vi "VolumeScan 1.4 - PointScan.vi"() -> ()   [LabVIEW 2020]
uses:
  <vilib>/vision/Image Controls.llb/IMAQ Image.ctl
  <vilib>/Utility/miscctls.llb/LVRowAndColumnTypeDef.ctl
  <vilib>/Utility/error.llb/DialogType.ctl
panel:
  out "Image":T1(plugin-control)
  in  "stop":bool
  in  "Zone":bool
  out "Status":string
  in  "Capture":bool
  in  "Tab Control":enum32{"Camera", "Display", "Saving"}(tab)
  in  "Pixels":dbl[][](array[numeric])
  in  "Threshold":dbl
  in  "Width":dbl
  in  "Band Start":dbl
  in  "ROI":dbl[](array[numeric])
  out "Node":dbl
  in  "Close camera":bool
  in  "Camera settings":bool
  in  "Camera settings table":i32(listbox)=-1
  in  "Open camera":bool
  in  "Display and panel":i32(ring) items=["2D Plot", "Default", "Graph"]
  in  "Path":path=path "G:/"
  in  "File Prefix":string="Prefix"
  in  "Save":T2(ring)
  in  "Shut Down":bool
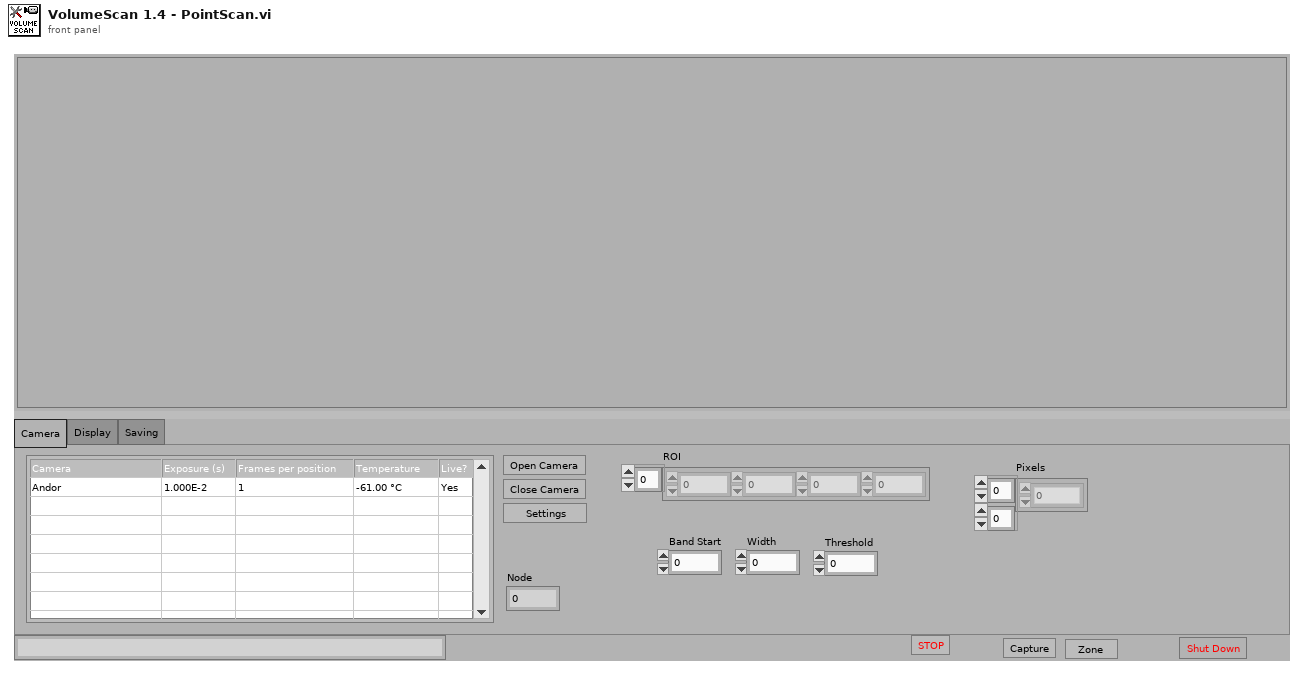
[diagram p1: front panel]
types:
  T1 = typedef "IMAQ Image.ctl" = refnum<image>
  T2 = enum16{"Don't save", "Save U16", "Save PNG", "Save TIFF"}
  T3 = cluster{"Driver":i32, "Camera settings":variant, "Update camera table":bool}
  T4 = typedef "LVRowAndColumnTypeDef.ctl" = cluster{"Row":i32, "Column":i32}
  T5 = enum8{"Enabled", "Disabled", "Disabled and Grayed Out"}
  T6 = cluster{enum16{"Image references", "Positions"}, "element data type":variant}
  T7 = enum16{"Initialize", "Shut down", "Set capture mode", "Set exposure", "Trigger and read", "Get status", "Other settings", "Idle", "Wake", "Save state"}
  T8 = enum32{"Invalid", "Standard", "Closed", "Hidden", "Minimized", "Maximized"}
  T9 = enum16{"Initialize", "Shut down", "Set capture mode", "Set exposure", "Trigger and read", "Get status", "Other settings"}
  T10 = cluster{"System OK?":bool, "Current exposure":dbl, "Temperature":dbl, "ROI":cluster{"X":u32, "X2":u32, "Y":u32, "Y2":u32}, "Binning":cluster{"X":u32, "Y":u32}}
  T11 = typedef "DialogType.ctl" = u16
  T12 = typedef "Image Type" = u32
  T13 = typedef "LVPoint32TypeDef.ctl" = cluster{"Horizontal":i32, "Vertical":i32}
  T14 = cluster{enum16{"Image references", "Positions"}, "Variant":variant}
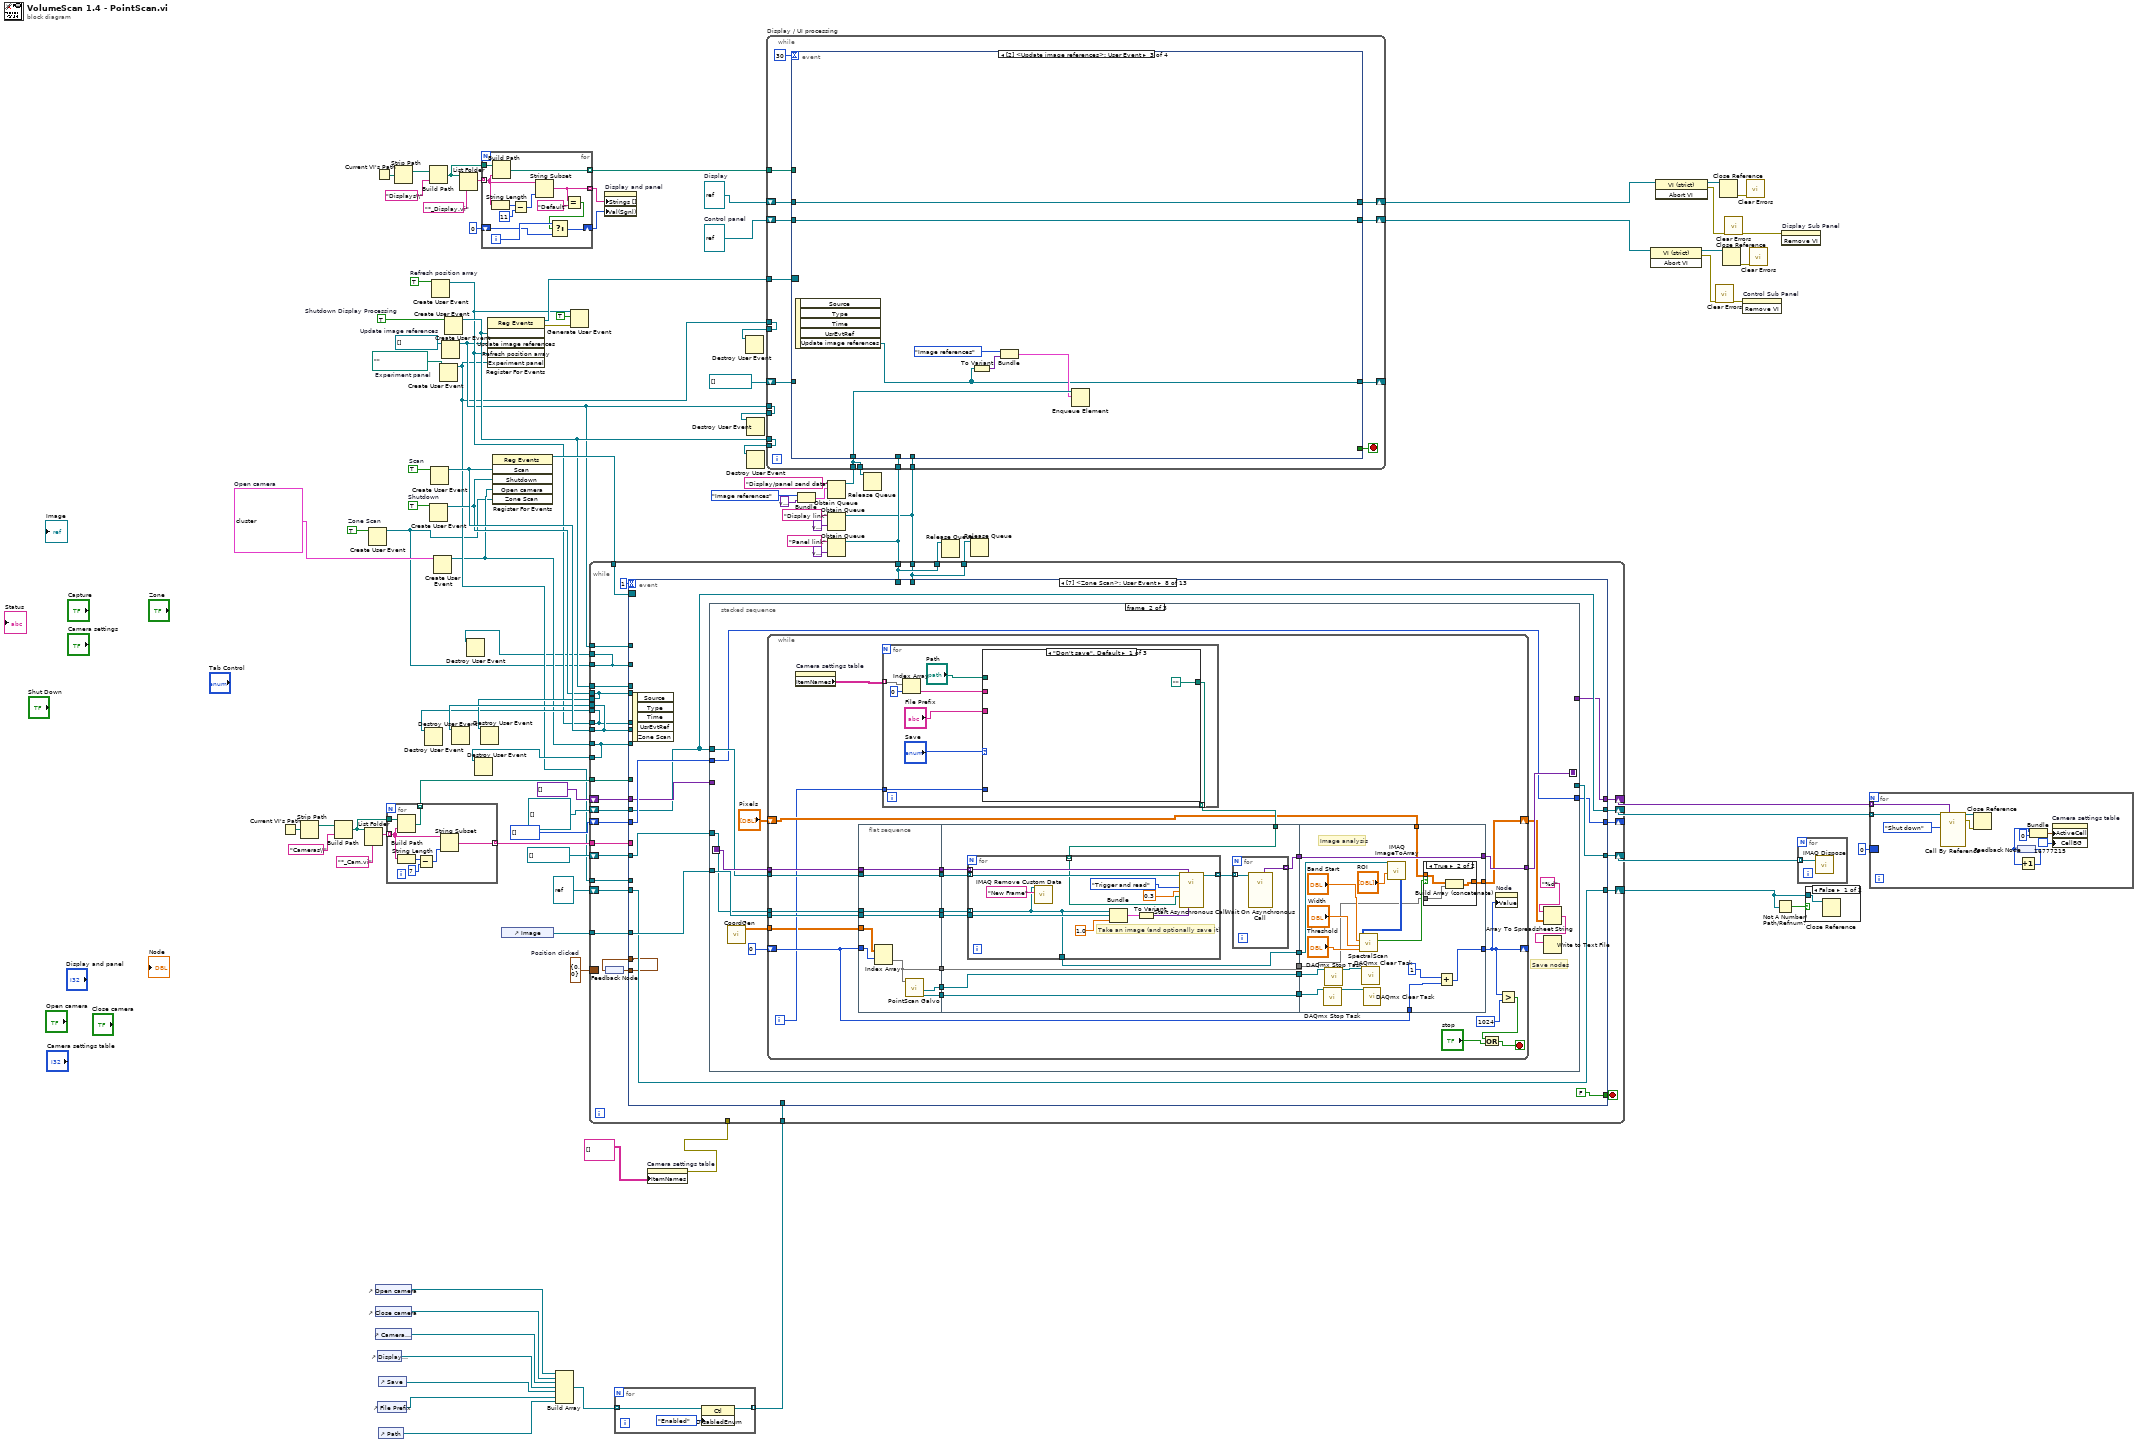
[diagram p0: block diagram]
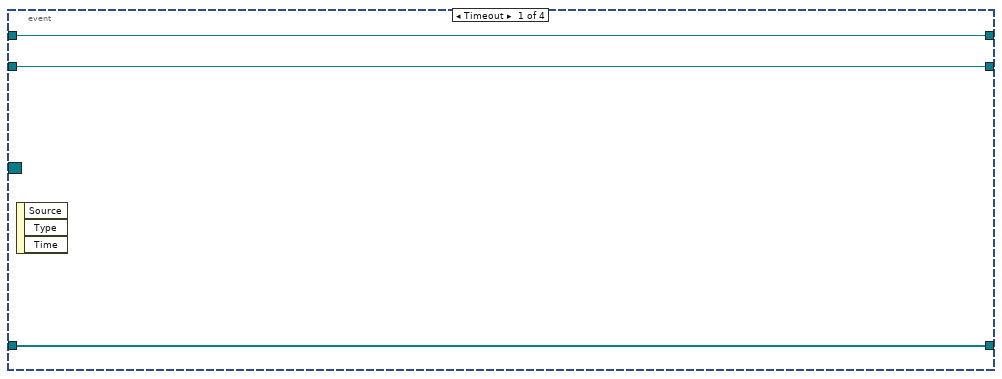
[diagram p3: hidden frame]
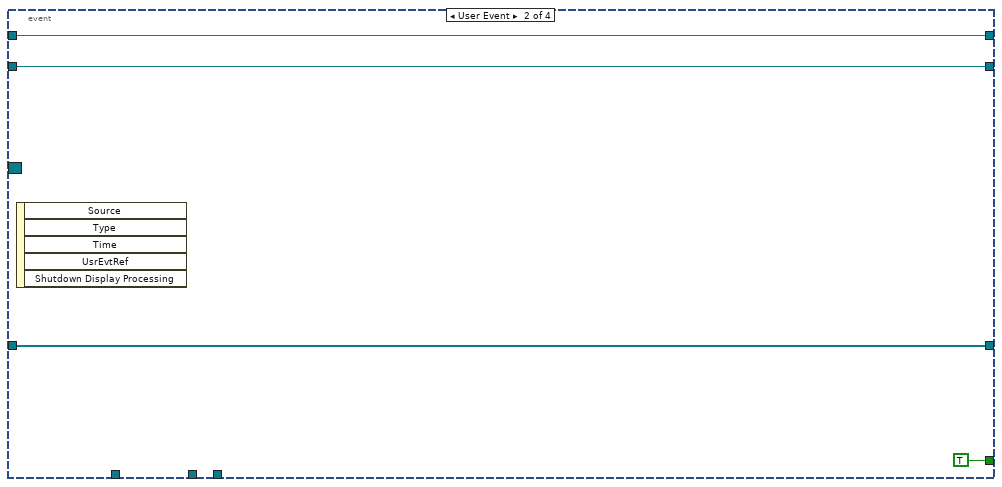
[diagram p4: hidden frame]
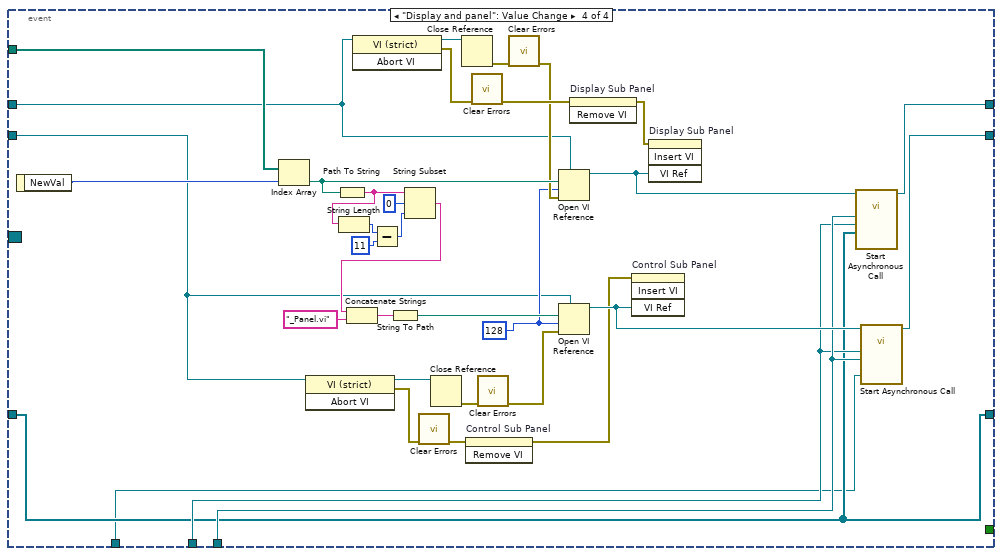
[diagram p5: hidden frame]
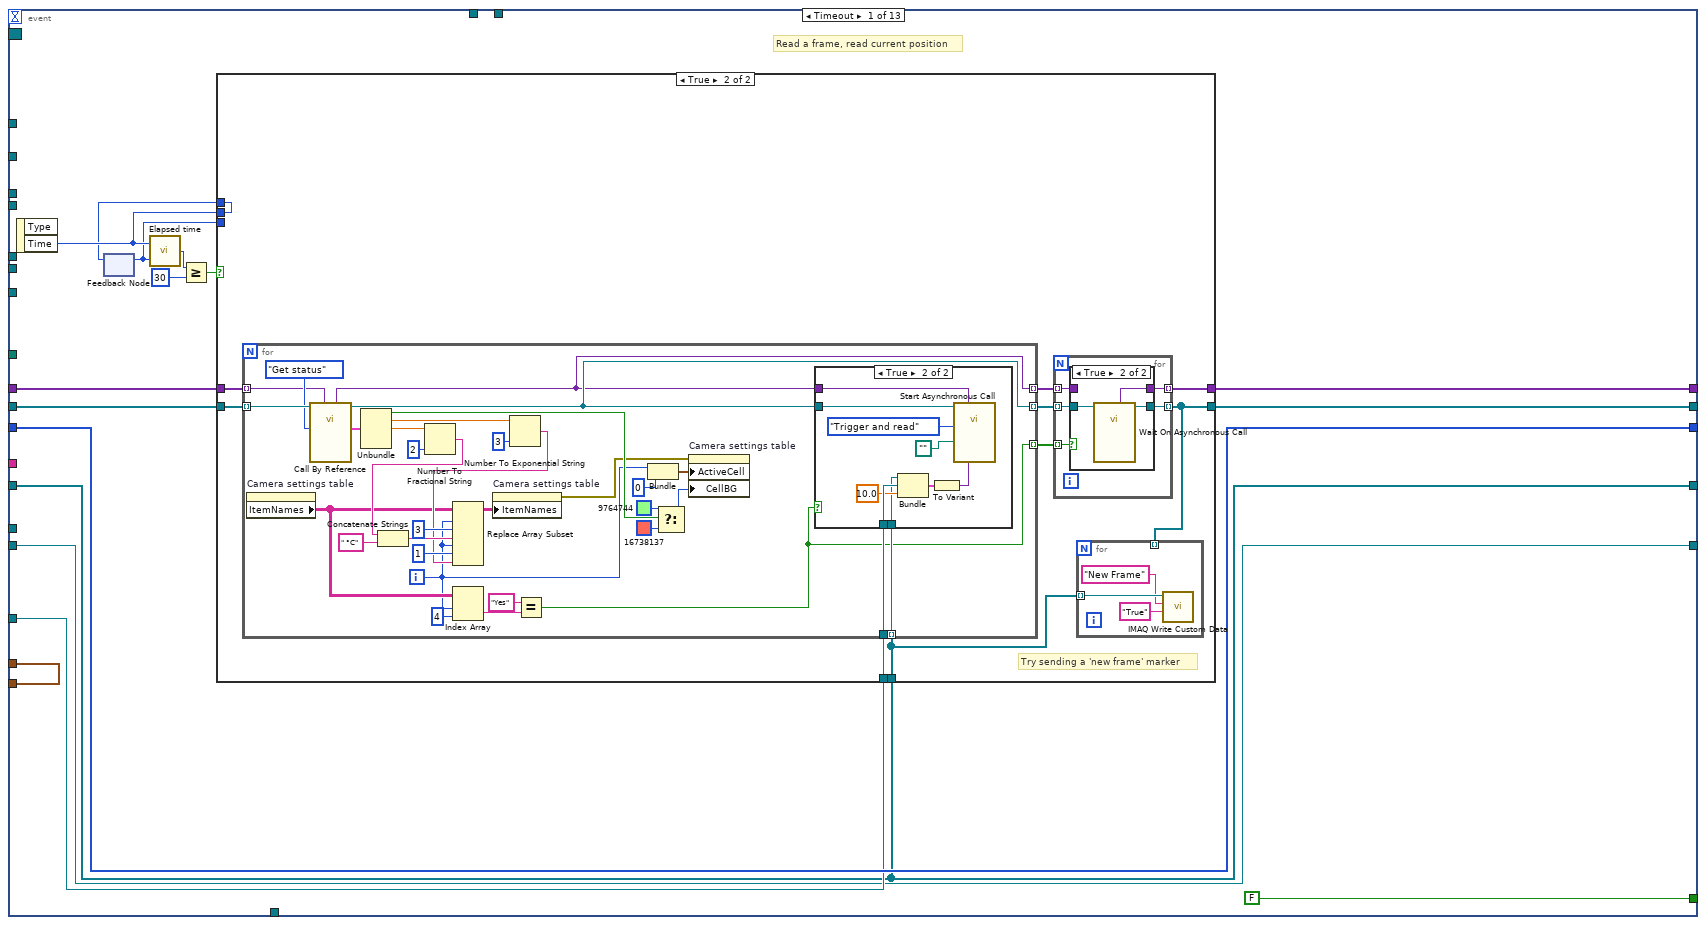
[diagram p6: hidden frame]
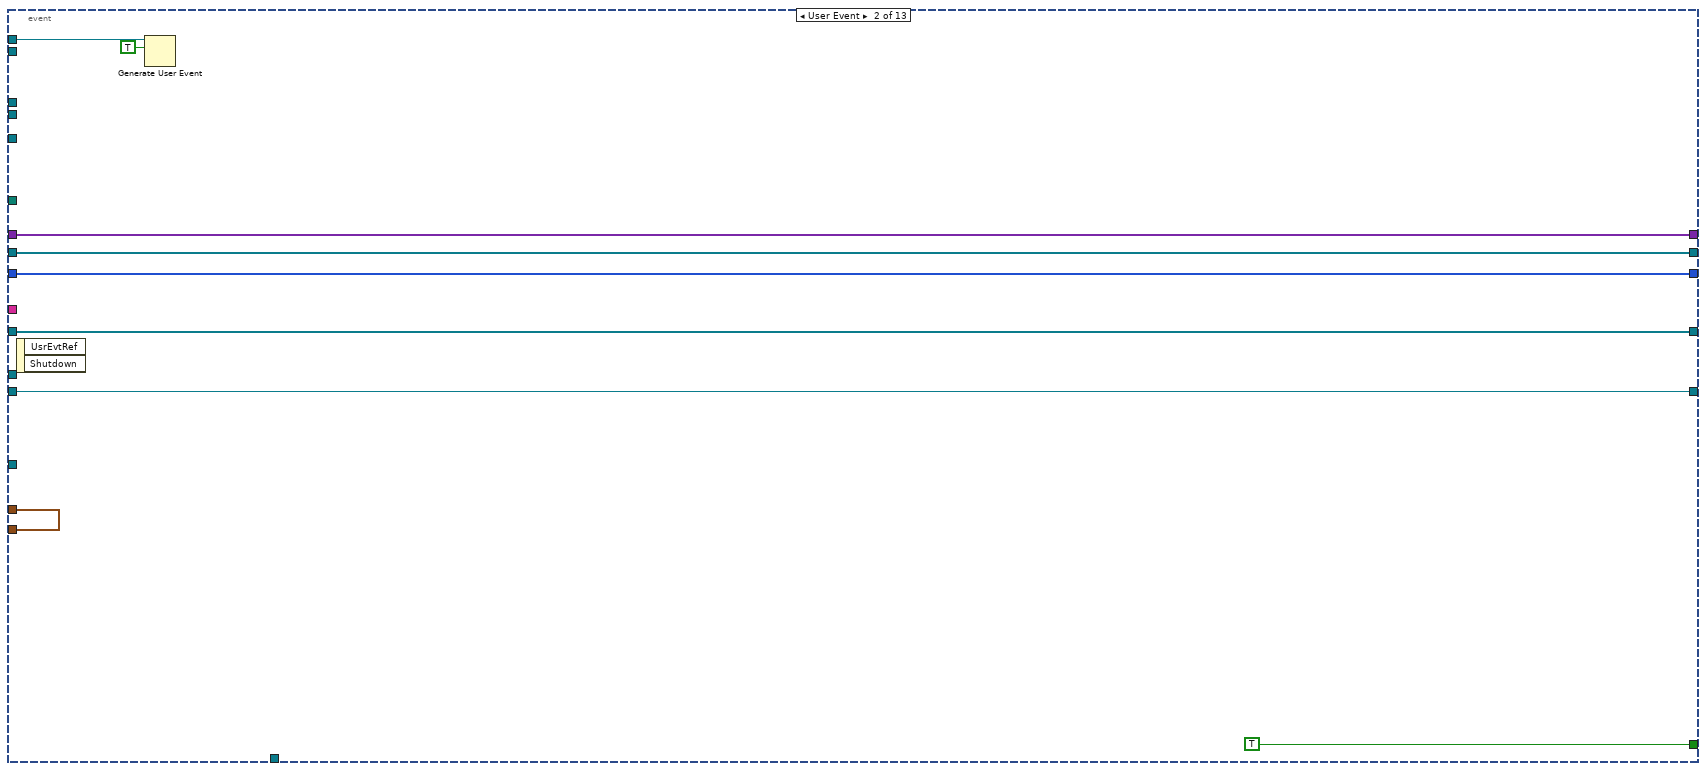
[diagram p10: hidden frame]
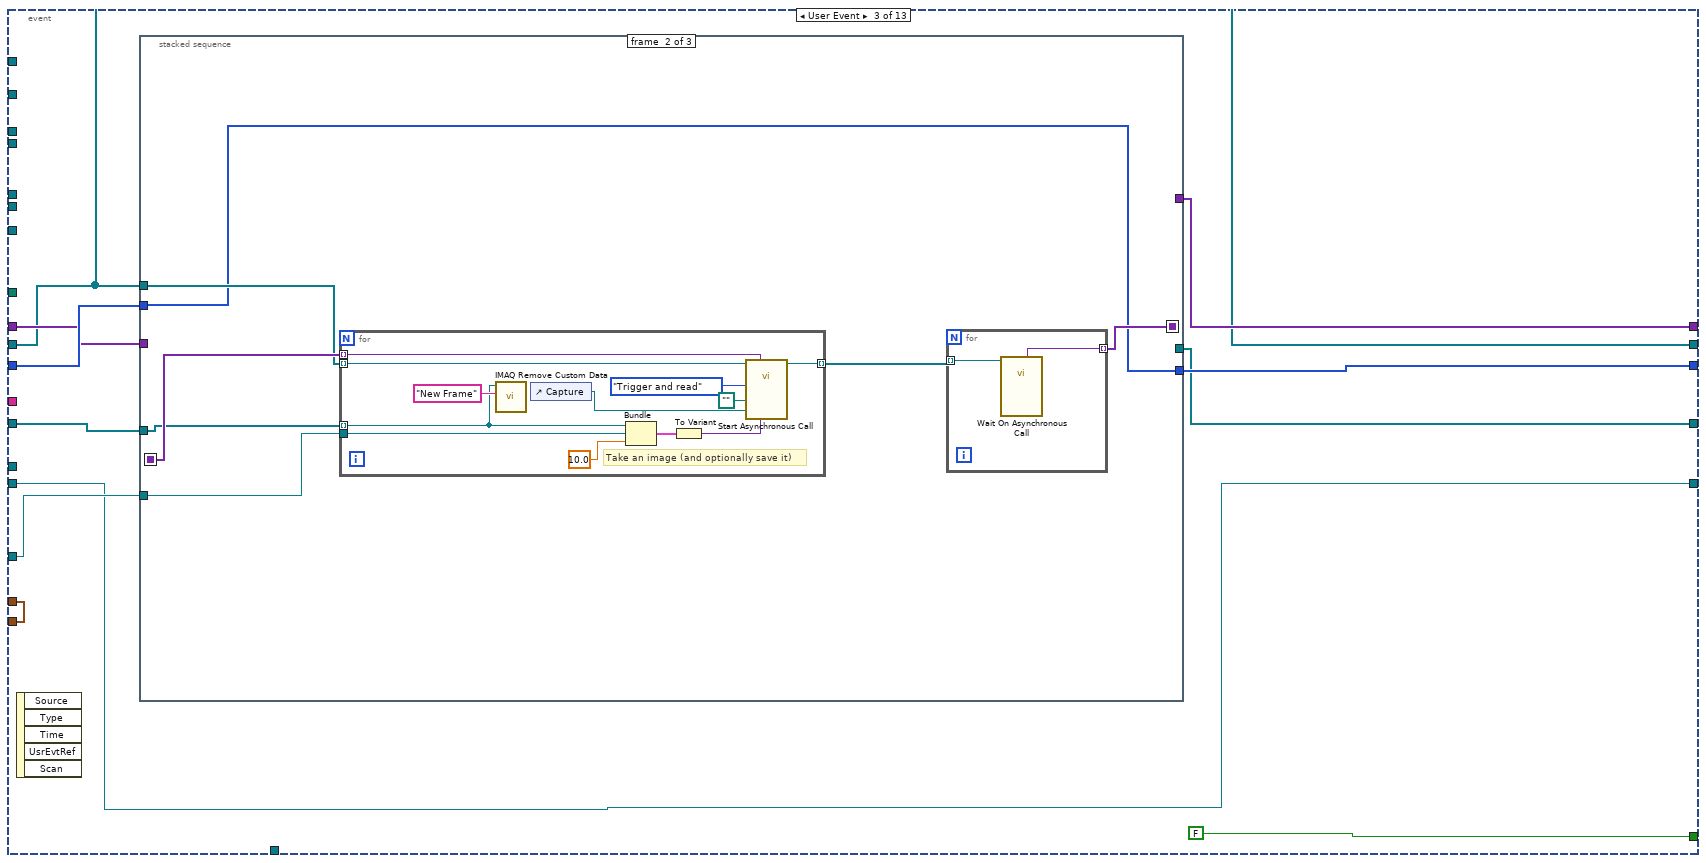
[diagram p11: hidden frame]
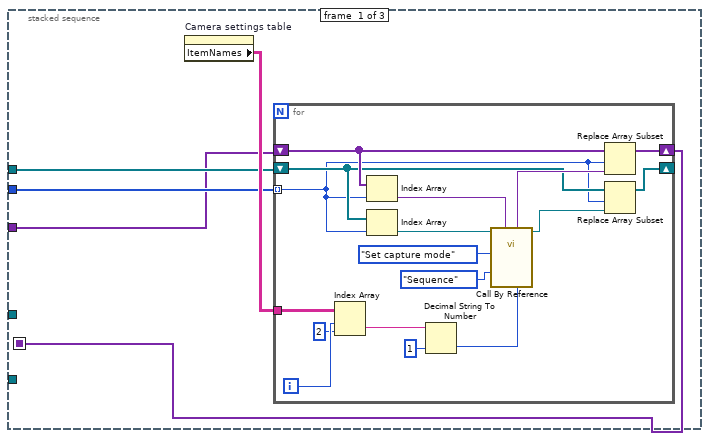
[diagram p12: hidden frame]
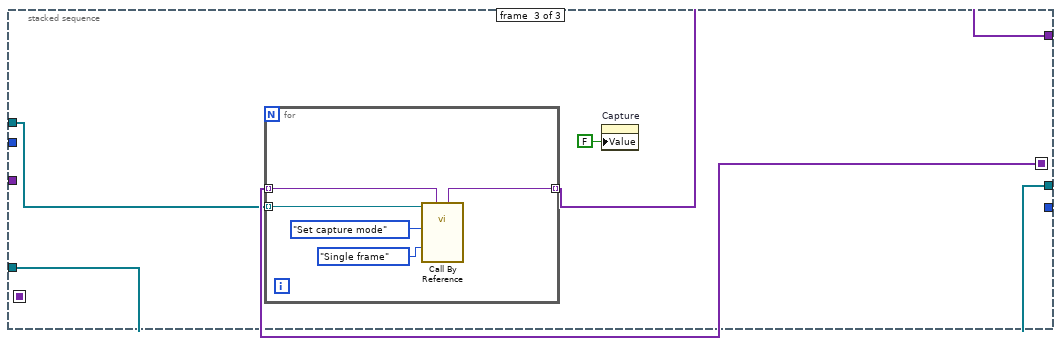
[diagram p13: hidden frame]
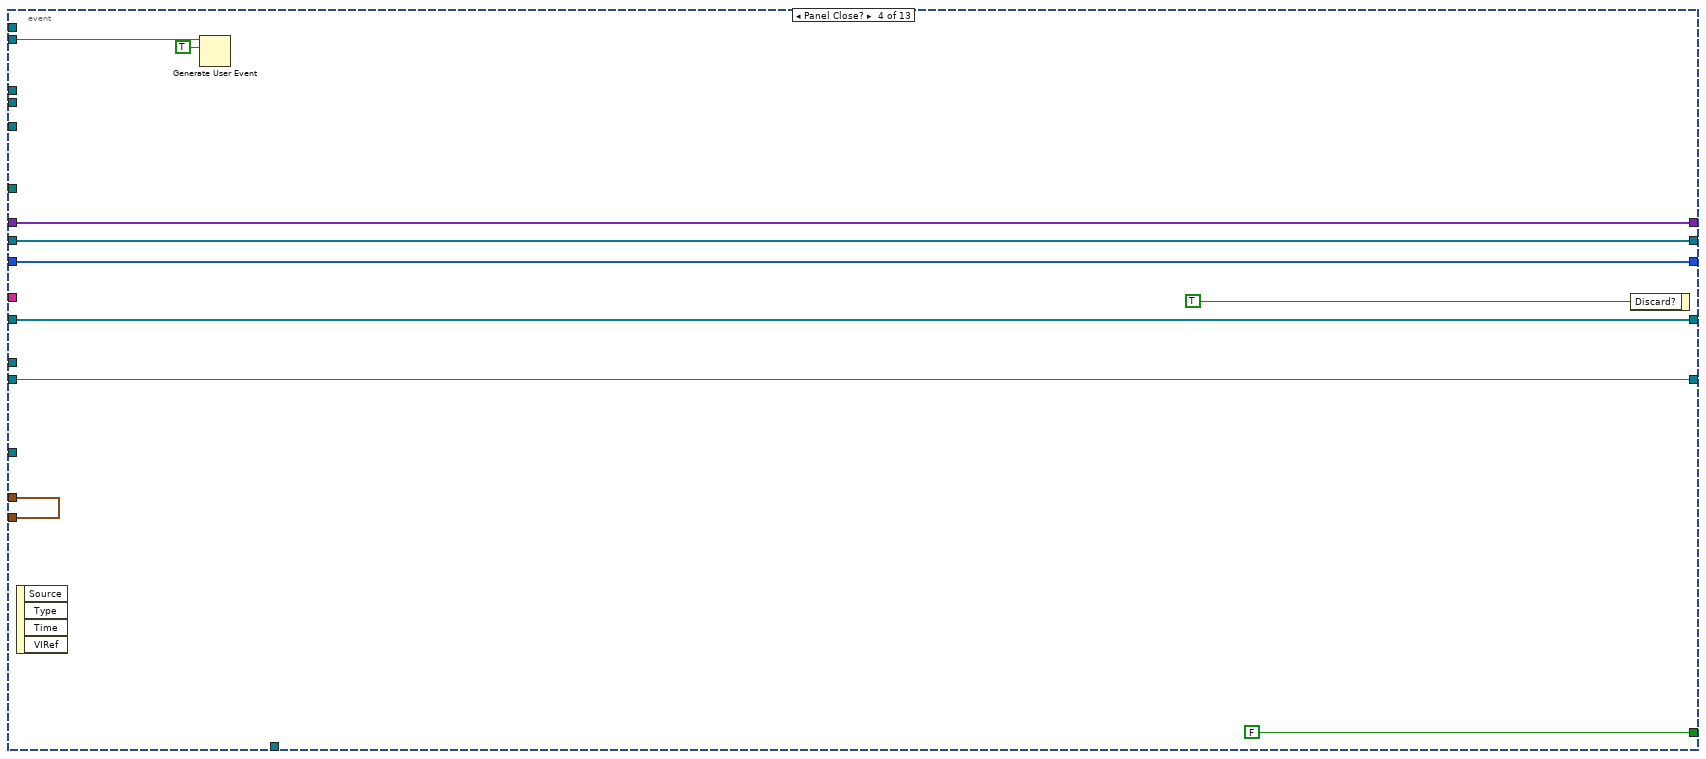
[diagram p14: hidden frame]
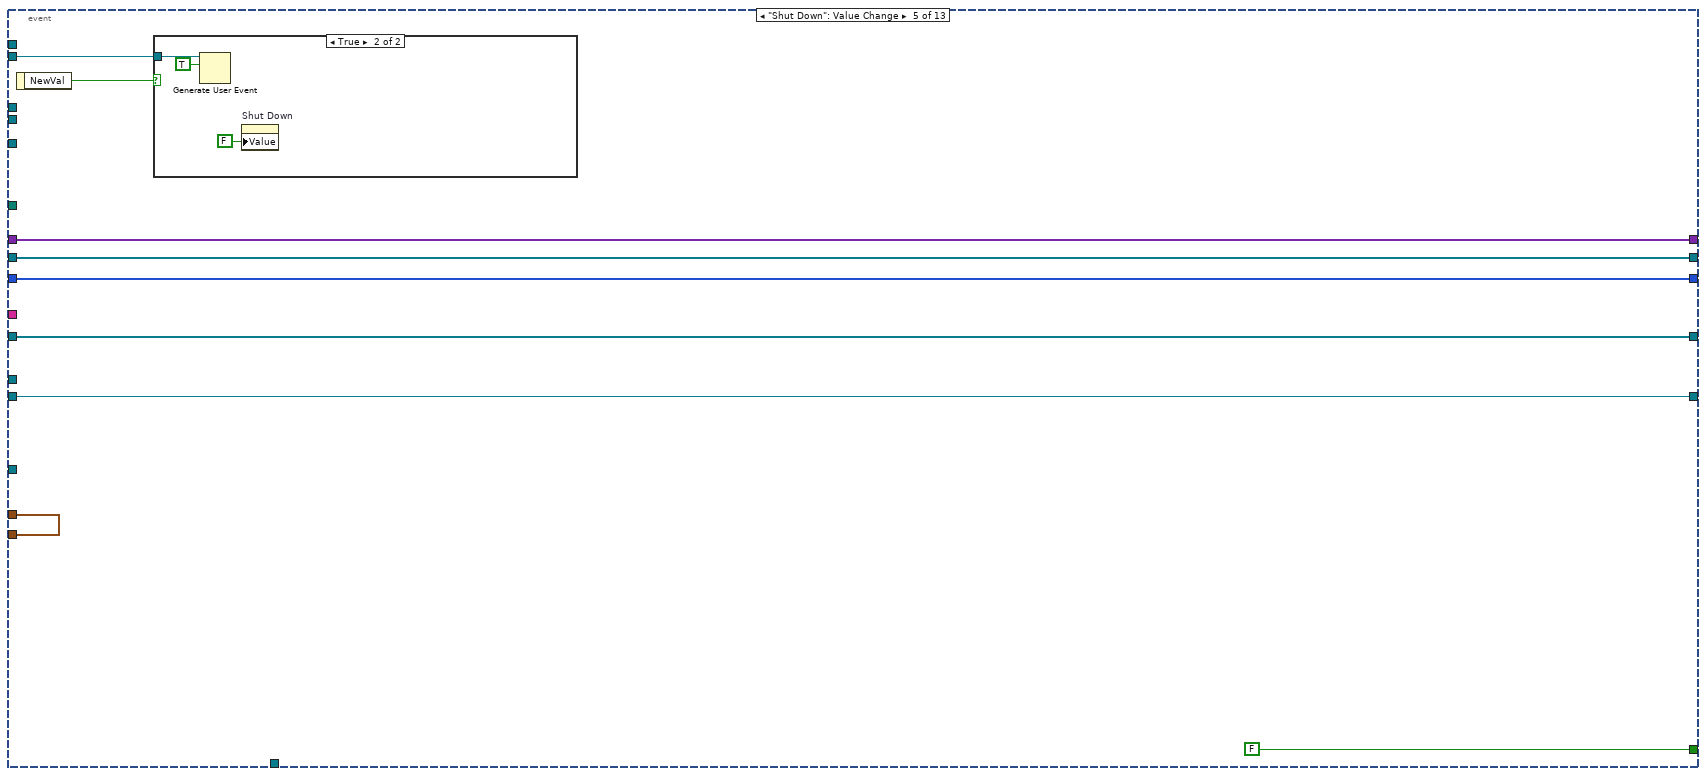
[diagram p15: hidden frame]
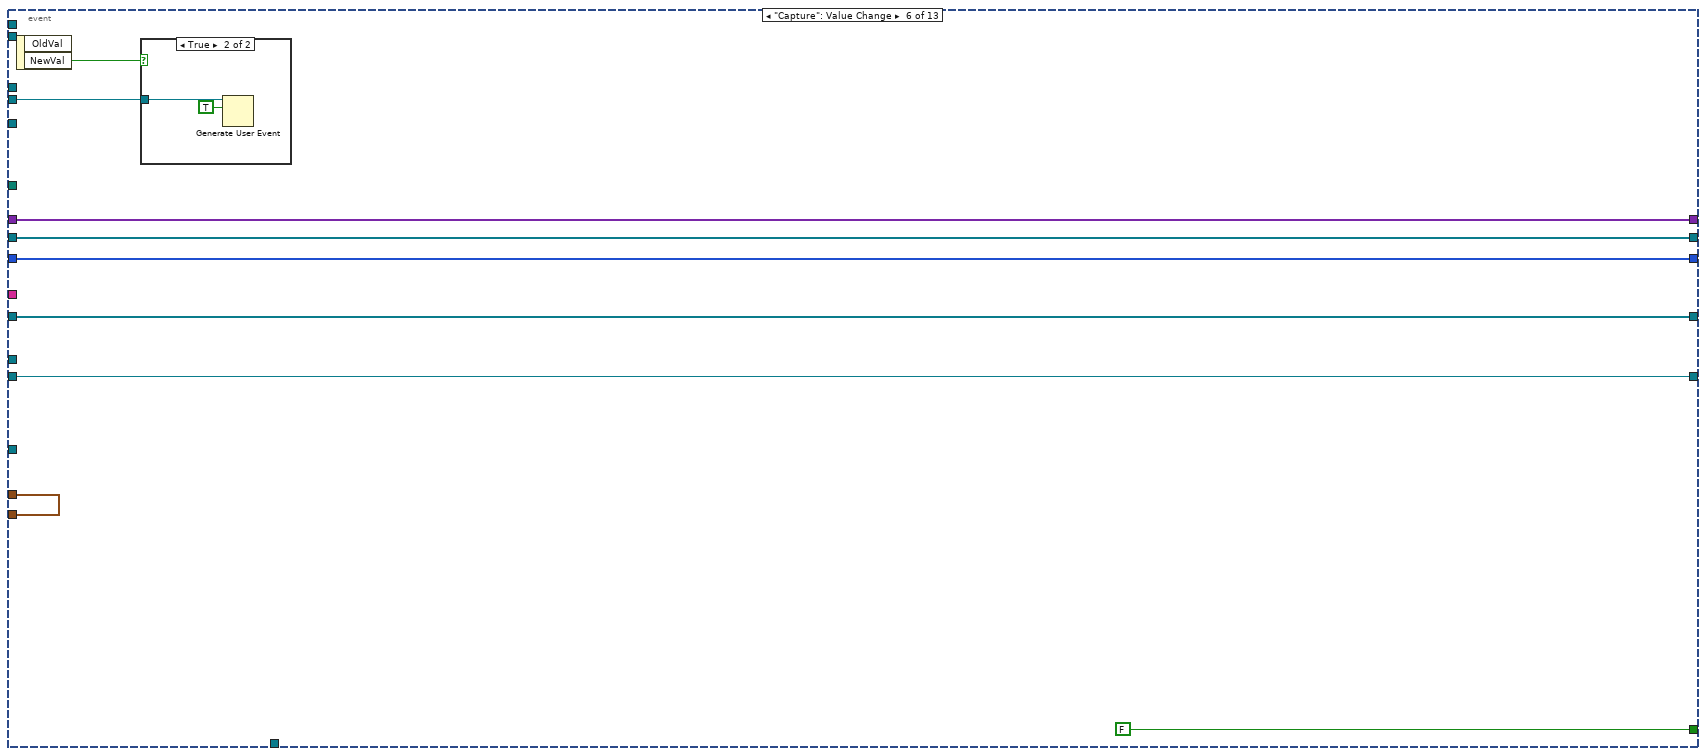
[diagram p17: hidden frame]
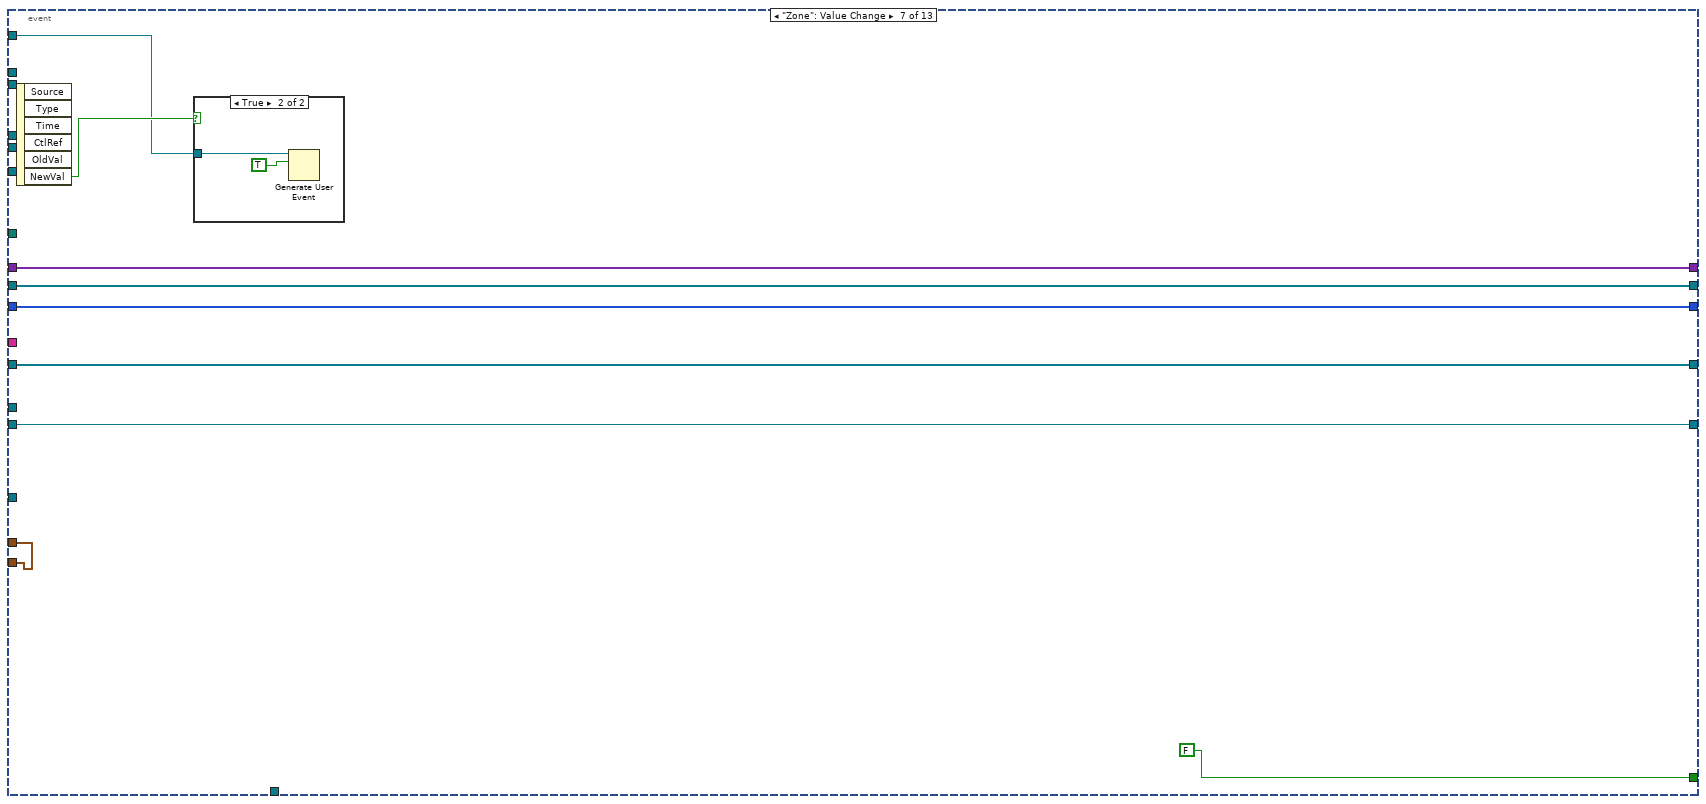
[diagram p19: hidden frame]
diagram:
  w6 = TRUE  # Zone Scan
  w12 = path ""  # Experiment panel
  w22 = T3 {"Driver"=0, "Camera settings"=variant, "Update camera table"=TRUE}  # Open camera
  w28 = TRUE  # Refresh position array
  w42 = refnum<vi> refnum  # Control panel
  w41 = refnum<vi> refnum  # Display
  w52 = T1[] []  # Update image references
  w79 = TRUE  # Shutdown Display Processing
  w80 = T4 {"Row"=0, "Column"=0}  # Position clicked
  w84 = TRUE  # Shutdown
  w97 = TRUE  # Scan
  n1 = Current VI's Path() -> (path=w94:path)
  n2 = Strip Path(path=w94) -> (stripped path=w93:path)  [unwired: 1 out]
  n3 = Build Path(base path=w93, name or relative path="Cameras\\") -> (appended path=w89:path)
  n4 = List Folder(path=w89, pattern="*_Cam.vi") -> (filenames=w90:string[])  [unwired: 2 in, 3 out]
  n5 = Create User Event(user event datatype=w6) -> (user event=w5:refnum<user-event>)  [unwired: 1 in, 1 out]
  n6 = Current VI's Path() -> (path=w68:path)
  n7 = control-ref of="Open camera"() -> (w50:refnum<vi>)
  n8 = control-ref of="Close camera"() -> (w49:refnum<vi>)
  n9 = control-ref of="Camera settings"() -> (w48:refnum<vi>)
  n10 = control-ref of="Display and panel"() -> (w47:refnum<vi>)
  n11 = control-ref of="File Prefix"() -> (w3:refnum<vi>)
  n12 = control-ref of="Save"() -> (w4:refnum<vi>)
  n13 = control-ref of="Path"() -> (w2:refnum<vi>)
  n14 = for {
    tunnel: w90 -> [w98] mode=indexing
    tunnel: [w100] -> w75 mode=indexing
    tunnel: w89 -> [w104]
    tunnel: [w103] -> w88 mode=indexing
    n15 = String Length(string=w98) -> (length=w102:i32)
    n16 = Build Path(base path=w104, name or relative path=w98) -> (appended path=w103:path)
    n17 = Subtract(x=w102, y=7) -> (x-y=w99:i32)
    n18 = String Subset(string=w98, length (rest)=w99) -> (substring=w100:string)  [unwired: 1 in]
  }
  n19 = Strip Path(path=w68) -> (stripped path=w67:path)  [unwired: 1 out]
  n20 = Build Path(base path=w67, name or relative path="Displays\\") -> (appended path=w62:path)
  n21 = Create User Event(user event datatype=w84) -> (user event=w82:refnum<user-event>)  [unwired: 1 in, 1 out]
  n22 = Create User Event(user event datatype=w97) -> (user event=w95:refnum<user-event>)  [unwired: 1 in, 1 out]
  n23 = Create User Event(user event datatype=w28) -> (user event=w25:refnum<user-event>)  [unwired: 1 in, 1 out]
  n24 = Create User Event(user event datatype=w22) -> (user event=w8:refnum<user-event>)  [unwired: 1 in, 1 out]
  n25 = Create User Event(user event datatype=w12) -> (user event=w10:refnum<user-event>)  [unwired: 1 in, 1 out]
  n26 = Create User Event(user event datatype=w52) -> (user event=w11:refnum<user-event>)  [unwired: 1 in, 1 out]
  n27 = Create User Event(user event datatype=w79) -> (user event=w76:refnum<user-event>)  [unwired: 1 in, 1 out]
  n28 = List Folder(path=w62, pattern="*_Display.vi") -> (filenames=w64:string[])  [unwired: 2 in, 3 out]
  n29 = for {
    tunnel: w64 -> [w105] mode=indexing
    tunnel: [w107] -> w70 mode=indexing
    shift-right: [w114] -> w69
    shift-left: 0 -> [w113]
    tunnel: w62 -> [w111]
    tunnel: [w110] -> w40 mode=indexing
    i -> [w115]
    n30 = String Length(string=w105) -> (length=w109:i32)
    n31 = Build Path(base path=w111, name or relative path=w105) -> (appended path=w110:path)
    n32 = Subtract(x=w109, y=11) -> (x-y=w106:i32)
    n33 = String Subset(string=w105, length (rest)=w106) -> (substring=w107:string)  [unwired: 1 in]
    n34 = Equal?(x=w107, y="Default") -> (x = y?=w112:bool)
    n35 = Select(t=w115, s=w112, f=w113) -> (s? t:f=w114:i32)
  }
  n36 = register-events(w76, w11, w25, w10) -> (reference out=w78:refnum<event-registration>, error out=w24:errorcluster)  [unwired: 2 in]
  n37 = register-events(w95, w82, w8, w5) -> (reference out=w96:refnum<event-registration>)  [unwired: 2 in, 1 out]
  n38 = control-ref of="Image"() -> (w85:refnum<vi>)
  n39 = Build Array(w50, w49, w48, w47, w4, w3, w2) -> (w46:refnum<vi>[])
  n40 = Generate User Event(user event=w25, event data cluster=TRUE ("event data"), error in=w24) -> ()  [unwired: 1 in, 2 out]
  n41 = property on="Display and panel" class="Ring (strict)"("Strings []"=w70, "Val(Sgnl)"=w69) -> ()  [unwired: 2 in, 2 out]
  n42 = for {
    tunnel: w46 -> [w119] mode=indexing
    tunnel: [w118] -> w45 mode=indexing
    n43 = property class="Ctl"(reference=w119, "DisabledEnum"=T5."Enabled" ("Disabled")) -> (reference out=w118:refnum<vi>)  [unwired: 1 in, 1 out]
  }
  n44 = property on="Camera settings table" class="MCListbox (strict)"("ItemNames"=string[][] [] ("Device setup")) -> (error out=w7:errorcluster)  [unwired: 2 in, 1 out]
  n45 = Bundle(enum16{"Image references", "Positions"}."Image references", "element data type"=variant) -> (w16:T6)  [unwired: 1 in]
  n46 = Obtain Queue(name (unnamed)="Display link", element data type=variant) -> (queue out=w43:refnum<queue>)  [unwired: 3 in, 2 out]
  n47 = Obtain Queue(name (unnamed)="Panel link", element data type=variant) -> (queue out=w44:refnum<queue>)  [unwired: 3 in, 2 out]
  n48 = while {
    tunnel: w96 -> [w146]
    tunnel: w95 -> [w139]
    shift-right: [w145] -> w87
    shift-left: refnum<vi>[] [] -> [w144]
    tunnel: w88 -> [w143]
    shift-right: [w142] -> w86
    shift-left: variant[] [] -> [w141]
    tunnel: w85 -> [w140]
    tunnel: [w139] -> w83
    tunnel: w82 -> [w138]
    tunnel: [w138] -> w81
    tunnel: w7 -> [_]
    border: w80 -> [_]
    tunnel: w76 -> [w135]
    tunnel: w75 -> [w134]
    shift-right: [w133] -> _
    shift-left: i32[] [] -> [w132]
    tunnel: w43 -> [w130]
    tunnel: w44 -> [w131]
    tunnel: [w131] -> w57
    tunnel: [w130] -> w56
    shift-right: [w128] -> w54
    shift-left: T1[] [] ("appended array") -> [w129]
    tunnel: w11 -> [w127]
    tunnel: w45 -> [w126]
    tunnel: w25 -> [w125]
    tunnel: [w125] -> w27
    tunnel: w8 -> [w124]
    tunnel: [w124] -> w23
    shift-right: [w122] -> w14
    shift-left: refnum<vi> refnum ("type specifier VI Refnum (for type only)") -> [w123]
    tunnel: w10 -> [w121]
    tunnel: w5 -> [w120]
    tunnel: [w120] -> w1
    stop <- w147 stop-if-true
    n49 = feedback #1() -> (w136:T4)
    n50 = event shown="[7] <Zone Scan>: User Event" {
      selector: w146 -> [_ _ _ _ _ _ _ _ _ _ _ _ _]
      dyn-events: _ -> [_ _ _ _ _ _ _ _ _ _ _ _ _]
      timeout: 1 -> [_ _ _ _ _ _ _ _ _ _ _ _ _]
      tunnel: [FALSE TRUE FALSE FALSE FALSE FALSE FALSE FALSE FALSE FALSE FALSE FALSE FALSE] -> w147
      tunnel: w139 -> [_ _ _ _ _ w334 _ _ _ _ _ _ _]
      tunnel: [w158 w238 w246 w312 w321 w332 w343 w355 w537 w618 w719 w818 w880] -> w145
      tunnel: w144 -> [w164 w238 w246 w312 w321 w332 w343 w355 w538 w579 w720 w820 w878]
      tunnel: w143 -> [_ _ _ _ _ _ _ _ w536 w617 _ _ _]
      tunnel: [w159 w239 w247 w313 w322 w331 w344 w351 w539 w619 w721 w816 w882] -> w142
      tunnel: w141 -> [w160 w239 w248 w313 w322 w331 w344 w358 w540 w620 w722 w815 w881]
      tunnel: w140 -> [w157 _ w250 _ _ _ _ w356 _ _ _ w810 _]
      tunnel: w138 -> [_ _ _ w310 w320 _ _ _ _ _ _ _ _]
      tunnel: [w162 w237 w242 w308 w318 w330 w339 w353 w542 w621 w724 w814 w899] -> w137
      tunnel: w136 -> [w162 w237 w242 w308 w318 w330 w339 w353 w542 w621 w724 w814 w899]
      tunnel: w135 -> [_ w235 _ _ _ _ _ _ _ _ _ _ _]
      tunnel: w134 -> [_ _ _ _ _ _ _ _ w541 w587 w723 _ _]
      tunnel: [w161 w234 w245 w307 w317 w329 w342 w349 w535 w616 w718 w813 w883] -> w133
      tunnel: w132 -> [w161 w234 w249 w307 w317 w329 w342 w359 w534 w615 w717 w813 w883]
      tunnel: w130 -> [_ _ _ _ _ _ _ _ _ w611 w713 _ _]
      tunnel: w131 -> [_ _ _ _ _ _ _ _ _ _ _ _ _]
      tunnel: w129 -> [w156 w233 w251 w306 w316 w328 w341 w357 w533 w614 w716 w811 w872]
      tunnel: [w156 w233 w244 w306 w316 w328 w341 w350 w532 w613 w715 w811 w872] -> w128
      tunnel: w127 -> [_ _ _ _ _ _ _ _ _ w612 w714 _ _]
      tunnel: w126 -> [_ _ _ _ _ _ _ _ _ _ _ _ _]
      tunnel: w125 -> [_ _ _ _ _ _ _ _ _ _ _ _ _]
      tunnel: w124 -> [_ _ _ _ _ _ _ _ w531 _ _ _ _]
      tunnel: w123 -> [w149 w232 w243 w305 w315 w327 w340 w354 w530 w580 w712 w812 w866]
      tunnel: [w149 w232 w243 w305 w315 w327 w340 w354 w530 w580 w712 w812 w866] -> w122
      tunnel: w121 -> [_ _ _ _ _ _ _ _ _ _ _ _ _]
      tunnel: w120 -> [_ _ _ _ _ _ w345 _ _ _ _ _ _]
      event Timeout {
        # "Read a frame, read current position"
        n51 = event-data() -> ("Time"=w152:u32)  [unwired: 1 in, 1 out]
        n52 = feedback #2() -> (w150:u32)  [unwired: 1 in]
        n53 = call "Elapsed time.vi"("Start time (ms)"=w150, "Current time (ms)"=w152) -> ("Elapsed time"=w155:u32)
        n54 = Greater Or Equal?(x=w155, y=u32 30) -> (x >= y?=w153:bool)
        n55 = case shown="True" w153 {
          tunnel: w164 -> [w166 w177]
          tunnel: w160 -> [w167 w170]
          tunnel: [w167 w176] -> w159
          tunnel: [w166 w174] -> w158
          tunnel: w157 -> [_ w172]
          tunnel: w156 -> [_ w173]
          tunnel: w152 -> [_ w175]
          tunnel: [w165 w175] -> w151
          tunnel: w150 -> [w165 _]
          frame False {
          }
          frame True {
            # "Try sending a 'new frame' marker"
            n56 = for {
              tunnel: w177 -> [w222] mode=indexing
              tunnel: [w198] -> w171 mode=indexing
              tunnel: w170 -> [w219] mode=indexing
              tunnel: w173 -> [w199] mode=indexing
              tunnel: w172 -> [w200]
              tunnel: [w192] -> w169 mode=indexing
              tunnel: [w191] -> w168 mode=indexing
              i -> [w196]
              n57 = property on="Camera settings table" class="MCListbox (strict)"() -> ("ItemNames"=w197:string[][])  [unwired: 2 in, 2 out]
              n58 = call-by-ref "?"(reference=w222, "Operation"=T7."Get status", "Camera-specific in"=w219) -> (reference out=w198:refnum<vi>, "Camera-specific out"=w191:variant, "Status"=w221:T10)  [unwired: 13 in, 1 out]
              n59 = Unbundle(w221) -> ("System OK?"=w213:bool, "Current exposure"=w202:dbl, "Temperature"=w210:dbl)  [unwired: 2 out]
              n60 = Number To Fractional String(number=w210, precision (6)=i16 2) -> (F-format string=w205:string)  [unwired: 2 in]
              n61 = Concatenate Strings(w205, " °C" ("string")) -> (w208:string)
              n62 = Index Array(array=w197, index (row)=w196, index (col)=4 ("disabled index (col)")) -> (element=w194:string)
              n63 = Number To Exponential String(number=w202, precision (6)=i16 3) -> (E-format string=w201:string)  [unwired: 2 in]
              n64 = Replace Array Subset(array=w197, new element #1=w208, index (row) #1=w196, index (col) #1=3 ("disabled index (col)"), new element #2=w201, index (row) #2=w196, index (col) #2=1 ("disabled index (col)")) -> (w212:string[][])
              n65 = property on="Camera settings table" class="MCListbox (strict)"("ItemNames"=w212) -> (error out=w207:errorcluster)  [unwired: 2 in, 1 out]
              n66 = Equal?(x="Yes", y=w194) -> (x = y?=w192:bool)
              n67 = Bundle(w196, 0) -> (w215:cluster{i32, i32})  [unwired: 1 in]
              n68 = Select(t=u32 9764744, s=w213, f=u32 16738137) -> (s? t:f=w216:u32)
              n69 = property on="Camera settings table" class="MCListbox (strict)"(error in=w207, "ActiveCell"=w215, "CellBG"=w216) -> ()  [unwired: 1 in, 2 out]
              n70 = case shown="True" w192 {
                tunnel: w191 -> [_ w223]
                tunnel: w200 -> [_ w227]
                tunnel: w199 -> [_ w225]
                tunnel: w198 -> [_ w224]
                frame False {
                }
                frame True {
                  n71 = Bundle("New Image"=w225, "Image"=w227, 10.0) -> (w231:cluster{"New Image":T1, "Image":refnum<vi>, dbl})  [unwired: 1 in]
                  n72 = To Variant(anything=w231) -> (Variant=w230:variant)
                  n73 = call-by-ref "Start Asynchronous Call"(reference=w224, "Operation"=T7."Trigger and read", "Camera-specific in"=w223, "Save path"=path "", "Image in"=w230) -> ()  [unwired: 11 in, 4 out]
                }
              }
            }
            n74 = for {
              tunnel: w171 -> [w182] mode=indexing
              tunnel: [w181] -> w176 mode=indexing
              tunnel: [w180] -> w174 mode=indexing
              tunnel: w169 -> [w179] mode=indexing
              tunnel: w168 -> [w178] mode=indexing
              n75 = case shown="True" w179 {
                tunnel: w182 -> [w184 w187]
                tunnel: [w183 w186] -> w181
                tunnel: [w184 w185] -> w180
                tunnel: w178 -> [w183 _]
                frame False {
                }
                frame True {
                  n76 = call-by-ref "Wait On Asynchronous Call"(reference=w187) -> (reference out=w185:refnum<vi>, "Camera-specific out"=w186:variant)  [unwired: 15 in, 2 out]
                }
              }
            }
            n77 = for {
              tunnel: w174 -> [_] mode=indexing
              tunnel: w173 -> [w190] mode=indexing
              n78 = call "IMAQ Write Custom Data"("Custom Data In"="True", "Key"="New Frame", "Image"=w190) -> ()  [unwired: 7 in, 2 out]
            }
          }
        }
        n79 = feedback-in #2(w151) -> ()
      }
      event User Event {
        n80 = event-data() -> ()  [unwired: 1 in, 2 out]
        n81 = Generate User Event(user event=w235, event data cluster=TRUE ("event data")) -> ()  [unwired: 2 in, 2 out]
      }
      event User Event {
        n82 = event-data() -> ()  [unwired: 1 in, 5 out]
        n83 = stacked-sequence {
          seq-local: [w254 _ _] -> [_ w278 _]
          seq-local: [_ w279 _] -> [_ _ w298]
          tunnel: w249 -> [w255 w274 _]
          tunnel: w251 -> [_ w275 w296]
          tunnel: w246 -> [w253 w277 w295]
          tunnel: w250 -> [_ w276 _]
          tunnel: [_ _ w297] -> w247
          tunnel: [_ _ w296] -> w244
          tunnel: w248 -> [w252 _ _]
          tunnel: [_ w274 _] -> w245
          frame #0 {
            n84 = property on="Camera settings table" class="MCListbox (strict)"() -> ("ItemNames"=w256:string[][])  [unwired: 2 in, 2 out]
            n85 = for {
              tunnel: w255 -> [w257] mode=indexing
              shift-right: [w269] -> w254
              shift-left: w252 -> [w270]
              shift-right: [w266] -> _
              shift-left: w253 -> [w265]
              tunnel: w256 -> [w263]
              i -> [w262]
              n86 = Index Array(array=w263, index (row)=w262, index (col)=2 ("disabled index (col)")) -> (element=w260:string)
              n87 = Index Array(array=w270, index=w257) -> (element=w271:variant)
              n88 = Index Array(array=w265, index=w257) -> (element=w267:refnum<vi>)
              n89 = Decimal String To Number(string=w260, default (0L)=u32 1 ("default (0 I32)")) -> (number=w258:u32)  [unwired: 1 in, 1 out]
              n90 = call-by-ref "?"(reference=w267, "Operation"=T7."Set capture mode", "Camera-specific in"=w271, "Capture mode"=enum16{"Single frame", "Sequence"}."Sequence", "Frames in sequence"=w258) -> (reference out=w264:refnum<vi>, "Camera-specific out"=w268:variant)  [unwired: 11 in, 2 out]
              n91 = Replace Array Subset(array=w270, new element=w268, index=w257) -> (w269:variant[])
              n92 = Replace Array Subset(array=w265, new element=w264, index=w257) -> (w266:refnum<vi>[])
            }
          }
          frame #1 {
            n93 = for {
              tunnel: w277 -> [w294] mode=indexing
              tunnel: w278 -> [w292] mode=indexing
              tunnel: w276 -> [w290]
              tunnel: w275 -> [w283] mode=indexing
              tunnel: [w287] -> w280 mode=indexing
              # "Take an image (and optionally save it)"
              n94 = call "IMAQ Remove Custom Data"("Key"="New Frame", "Image"=w283) -> ()  [unwired: 7 in, 3 out]
              n95 = control-ref of="Capture"() -> (w285:refnum<vi>)
              n96 = Bundle("New Image"=w283, "Image"=w290, 10.0) -> (w291:cluster{"New Image":T1, "Image":refnum<vi>, dbl})  [unwired: 1 in]
              n97 = To Variant(anything=w291) -> (Variant=w288:variant)
              n98 = call-by-ref "Start Asynchronous Call"(reference=w294, "Operation"=T7."Trigger and read", "Camera-specific in"=w292, "Save path"=path "", "Capture button"=w285, "Image in"=w288) -> (reference out=w287:refnum<vi>)  [unwired: 10 in, 3 out]
            }
            n99 = for {
              tunnel: w280 -> [w282] mode=indexing
              tunnel: [w281] -> w279 mode=indexing
              n100 = call-by-ref "Wait On Asynchronous Call"(reference=w282) -> ("Camera-specific out"=w281:variant)  [unwired: 15 in, 3 out]
            }
          }
          frame #2 {
            n101 = for {
              tunnel: w295 -> [w303] mode=indexing
              tunnel: w298 -> [w301] mode=indexing
              tunnel: [w300] -> w297 mode=indexing
              n102 = call-by-ref "?"(reference=w303, "Operation"=T7."Set capture mode", "Camera-specific in"=w301, "Capture mode"=enum16{"Single frame", "Sequence"}."Single frame") -> ("Camera-specific out"=w300:variant)  [unwired: 12 in, 3 out]
            }
            n103 = property on="Capture" class="Bool (strict)"("Value"=FALSE ("Capture")) -> ()  [unwired: 2 in, 2 out]
          }
        }
      }
      event Panel Close? {
        n104 = event-data() -> ()  [unwired: 1 in, 4 out]
        n105 = Generate User Event(user event=w310, event data cluster=TRUE ("event data")) -> ()  [unwired: 2 in, 2 out]
        n106 = event-data("Discard?"=TRUE) -> ()  [unwired: 1 in, 1 out]
      }
      event "Shut Down": Value Change {
        n107 = event-data() -> ("NewVal"=w319:bool)  [unwired: 1 in]
        n108 = case shown="True" w319 {
          tunnel: w320 -> [_ w326]
          frame False {
          }
          frame True {
            n109 = Generate User Event(user event=w326, event data cluster=TRUE ("event data")) -> ()  [unwired: 2 in, 2 out]
            n110 = property on="Shut Down" class="Bool (strict)"("Value"=FALSE ("Shut Down")) -> ()  [unwired: 2 in, 2 out]
          }
        }
      }
      event "Capture": Value Change {
        n111 = event-data() -> ("NewVal"=w335:bool)  [unwired: 1 in, 1 out]
        n112 = case shown="True" w335 {
          tunnel: w334 -> [_ w337]
          frame False {
          }
          frame True {
            n113 = Generate User Event(user event=w337, event data cluster=TRUE ("event data")) -> ()  [unwired: 2 in, 2 out]
          }
        }
      }
      event "Zone": Value Change {
        n114 = event-data() -> ("NewVal"=w346:bool)  [unwired: 1 in, 5 out]
        n115 = case shown="True" w346 {
          tunnel: w345 -> [_ w347]
          frame False {
          }
          frame True {
            n116 = Generate User Event(user event=w347, event data cluster=TRUE ("event data")) -> ()  [unwired: 2 in, 2 out]
          }
        }
      }
      event User Event {
        n117 = event-data() -> ()  [unwired: 1 in, 5 out]
        n118 = stacked-sequence {
          seq-local: [w362 _ _] -> [_ w392 _]
          seq-local: [_ w393 _] -> [_ _ w524]
          tunnel: w359 -> [w363 w388 _]
          tunnel: w357 -> [_ w389 w522]
          tunnel: w355 -> [w361 w391 w521]
          tunnel: w356 -> [_ w390 _]
          tunnel: [_ _ w523] -> w351
          tunnel: [_ _ w522] -> w350
          tunnel: w358 -> [w360 _ _]
          tunnel: [_ w388 _] -> w349
          frame #0 {
            n119 = property on="Camera settings table" class="MCListbox (strict)"() -> ("ItemNames"=w364:string[][])  [unwired: 2 in, 2 out]
            n120 = for {
              tunnel: w363 -> [w365] mode=indexing
              shift-right: [w377] -> w362
              shift-left: w360 -> [w378]
              shift-right: [w374] -> _
              shift-left: w361 -> [w373]
              tunnel: w364 -> [w371]
              i -> [w370]
              n121 = Index Array(array=w371, index (row)=w370, index (col)=2 ("disabled index (col)")) -> (element=w368:string)
              n122 = Index Array(array=w378, index=w365) -> (element=w379:variant)
              n123 = Index Array(array=w373, index=w365) -> (element=w375:refnum<vi>)
              n124 = Decimal String To Number(string=w368, default (0L)=u32 1 ("default (0 I32)")) -> (number=w366:u32)  [unwired: 1 in, 1 out]
              n125 = call-by-ref "?"(reference=w375, "Operation"=T7."Set capture mode", "Camera-specific in"=w379, "Capture mode"=enum16{"Single frame", "Sequence"}."Sequence", "Frames in sequence"=w366) -> (reference out=w372:refnum<vi>, "Camera-specific out"=w376:variant)  [unwired: 11 in, 2 out]
              n126 = Replace Array Subset(array=w378, new element=w376, index=w365) -> (w377:variant[])
              n127 = Replace Array Subset(array=w373, new element=w372, index=w365) -> (w374:refnum<vi>[])
            }
          }
          frame #1 {
            # "Save nodes"
            n128 = call "CoordGen.vi"() -> ("Coord"=w382:dbl[][])  [unwired: 11 in]
            n129 = while {
              tunnel: [w418] -> w393
              tunnel: w392 -> [w417]
              tunnel: w391 -> [w416]
              tunnel: w390 -> [w415]
              tunnel: w389 -> [w414]
              shift-right: [w401] -> _
              shift-left: 0 -> [w403]
              shift-right: [w399] -> w385
              shift-left: "Pixels" -> [w400]
              tunnel: w382 -> [w394]
              i -> [w395]
              stop <- w396 stop-if-true
              n130 = property on="Camera settings table" class="MCListbox (strict)"() -> ("ItemNames"=w412:string[][])  [unwired: 2 in, 2 out]
              n131 = flat-sequence {
                tunnel: w414 -> [w469]
                tunnel: w415 -> [w470]
                tunnel: w416 -> [w471]
                tunnel: w417 -> [w472]
                tunnel: [w472] -> w422
                tunnel: [w471] -> w421
                tunnel: [w470] -> w420
                tunnel: [w469] -> w419
                tunnel: [w467] -> w411
                tunnel: w403 -> [w468]
                tunnel: [w466] -> w406
                tunnel: [w465] -> w404
                tunnel: w394 -> [w464]
                tunnel: w422 -> [w481]
                tunnel: w421 -> [w480]
                tunnel: w420 -> [w479]
                tunnel: w419 -> [w478]
                tunnel: w413 -> [w477]
                tunnel: w411 -> [w476]
                tunnel: [w482] -> w410
                tunnel: [w476] -> w409
                tunnel: [w475] -> w408
                tunnel: [w474] -> w407
                tunnel: w406 -> [w474]
                tunnel: [w473] -> w405
                tunnel: w404 -> [w473]
                tunnel: [w515] -> w418
                tunnel: w410 -> [w515]
                tunnel: w409 -> [w514]
                tunnel: w408 -> [w512]
                tunnel: w407 -> [w509]
                tunnel: w405 -> [w501]
                tunnel: w403 -> [w508]
                tunnel: [w507] -> w401
                tunnel: w400 -> [w500]
                tunnel: [w499] -> w399
                frame #0 {
                  n132 = Index Array(array=w464, index (row)=w468) -> (element=w465:dbl[])  [unwired: 1 in]
                  n133 = call "PointScan Galvo.vi"("Input Coords"=w465) -> ("AI out"=w466:refnum<k21>, "AO out"=w467:refnum<k21>)  [unwired: 9 in]
                }
                frame #1 {
                  n134 = for {
                    tunnel: w480 -> [w497] mode=indexing
                    tunnel: w481 -> [w495] mode=indexing
                    tunnel: w479 -> [w493]
                    tunnel: w478 -> [w486] mode=indexing
                    tunnel: [w491] -> w483 mode=indexing
                    tunnel: w477 -> [w489] mode=indexing
                    tunnel: [w486] -> w475
                    # "Take an image (and optionally save it)"
                    n135 = call "IMAQ Remove Custom Data"("Key"="New Frame", "Image"=w486) -> ()  [unwired: 7 in, 3 out]
                    n136 = Bundle("New Image"=w486, "Image"=w493, 1.0) -> (w494:cluster{"New Image":T1, "Image":refnum<vi>, dbl})  [unwired: 1 in]
                    n137 = To Variant(anything=w494) -> (Variant=w487:variant)
                    n138 = call-by-ref "Start Asynchronous Call"(reference=w497, "Operation"=T7."Trigger and read", "Camera-specific in"=w495, "Exposure time (s)"=0.3, "Save path"=w489, "Image in"=w487) -> (reference out=w491:refnum<vi>)  [unwired: 10 in, 3 out]
                  }
                  n139 = for {
                    tunnel: w483 -> [w485] mode=indexing
                    tunnel: [w484] -> w482 mode=indexing
                    n140 = call-by-ref "Wait On Asynchronous Call"(reference=w485) -> ("Camera-specific out"=w484:variant)  [unwired: 15 in, 3 out]
                  }
                }
                frame #2 {
                  # "Image analysis"
                  n141 = call <vilib>:"DAQmx Stop Task.vi"("task/channels in"=w509) -> ("task out"=w510:refnum<k21>)  [unwired: 13 in, 1 out]
                  n142 = call <vilib>:"DAQmx Stop Task.vi"("task/channels in"=w514) -> ("task out"=w513:refnum<k21>)  [unwired: 13 in, 1 out]
                  n143 = call <vilib>:"DAQmx Clear Task.vi"("task in"=w513) -> ()  [unwired: 14 in, 1 out]
                  n144 = call <vilib>:"DAQmx Clear Task.vi"("task in"=w510) -> ()  [unwired: 14 in, 1 out]
                  n145 = call "IMAQ ImageToArray"("Optional Rectangle"="ROI", "Image"=w512) -> ("Image Pixels (U16)"=w511:u16[][])  [unwired: 2 in, 4 out]
                  n146 = call "SpectralScan.vi"("Threshold"="Threshold", "Band Size"="Width", "Start Band"="Band Start", "Array"=w511) -> ("Signal?"=w506:bool)  [unwired: 6 in, 1 out]
                  n147 = case shown="True" w506 {
                    tunnel: w501 -> [_ w519]
                    tunnel: w500 -> [w516 w518]
                    tunnel: [w516 w517] -> w499
                    frame False {
                    }
                    frame True {
                      n148 = Build Array (concatenate)(w518, w519) -> (w517:dbl[][])
                    }
                  }
                  n149 = Add(x=1, y=w508) -> (x+y=w507:i32)
                }
              }
              n150 = for {
                tunnel: w412 -> [w430] mode=indexing
                tunnel: [w427] -> w413 mode=indexing
                tunnel: w395 -> [w423]
                n151 = Index Array(array=w430, index=0) -> (element=w429:string)
                n152 = case shown="\"Don't save\", Default" "Save" {
                  tunnel: "Path" -> [_ w443 w459]
                  tunnel: "File Prefix" -> [_ w437 w454]
                  tunnel: [path "" w439 w455] -> w427
                  tunnel: w429 -> [_ w435 w452]
                  tunnel: w423 -> [_ _ w448]
                  frame "Don't save", Default {
                  }
                  frame "Save TIFF" {
                    n153 = call <vilib>:"Check if File or Folder Exists.vi"("path"=w443) -> ("file or folder exists?"=w442:bool, "dup path"=w441:path)  [unwired: 8 in, 1 out]
                    n154 = Tick Count (ms)() -> (millisecond timer value=w438:u32)
                    n155 = case shown="False" w442 {
                      tunnel: w441 -> [w446 w447]
                      tunnel: [w445 w447] -> w440
                      frame False {
                        n156 = Create Folder(path (use dialog)=w446) -> (created path=w445:path)  [unwired: 2 in, 2 out]
                      }
                      frame True {
                      }
                    }
                    n157 = Number To Decimal String(number=w438) -> (decimal integer string=w433:string)  [unwired: 1 in]
                    n158 = Concatenate Strings(w437, "_", w435, "_t=", w433, ".tif") -> (w444:string)
                    n159 = Build Path(base path=w440, name or relative path=w444) -> (appended path=w439:path)
                  }
                  frame "Save U16" {
                    n160 = call <vilib>:"Check if File or Folder Exists.vi"("path"=w459) -> ("file or folder exists?"=w458:bool, "dup path"=w457:path)  [unwired: 8 in, 1 out]
                    n161 = case shown="False" w458 {
                      tunnel: w457 -> [w462 w463]
                      tunnel: [w461 w463] -> w456
                      frame False {
                        n162 = Create Folder(path (use dialog)=w462) -> (created path=w461:path)  [unwired: 2 in, 2 out]
                      }
                      frame True {
                      }
                    }
                    n163 = Number To Decimal String(number=w448) -> (decimal integer string=w450:string)  [unwired: 1 in]
                    n164 = Concatenate Strings(w454, "_", w452, "_t=", w450, ".U16") -> (w460:string)
                    n165 = Build Path(base path=w456, name or relative path=w460) -> (appended path=w455:path)
                  }
                }
              }
              n166 = property on="Node" class="DigNum (strict)"("Value"=w401) -> ()  [unwired: 2 in, 2 out]
              n167 = Greater?(x=w401, y=1024) -> (0:w398:bool)
              n168 = Or(x=w398, y="stop") -> (x .or. y?=w396:bool)
            }
            n169 = Array To Spreadsheet String(array=w385, 3:"%d") -> (spreadsheet string=w383:string)  [unwired: 1 in]
            n170 = Write to Text File(text=w383) -> ()  [unwired: 3 in, 3 out]
          }
          frame #2 {
            n171 = for {
              tunnel: w521 -> [w528] mode=indexing
              tunnel: w524 -> [w526] mode=indexing
              tunnel: [w525] -> w523 mode=indexing
              n172 = call-by-ref "?"(reference=w528, "Operation"=T7."Set capture mode", "Camera-specific in"=w526, "Capture mode"=enum16{"Single frame", "Sequence"}."Single frame") -> ("Camera-specific out"=w525:variant)  [unwired: 12 in, 3 out]
            }
            n173 = property on="Zone" class="Bool (strict)"("Value"=FALSE ("Capture")) -> ()  [unwired: 2 in, 2 out]
          }
        }
      }
      event "Open camera": Value Change {
        n174 = event-data() -> ("NewVal"=w543:bool)  [unwired: 1 in]
        n175 = case shown="True" w543 {
          tunnel: w541 -> [_ w559]
          tunnel: w540 -> [w548 w558]
          tunnel: w538 -> [w547 w557]
          tunnel: [w548 w556] -> w539
          tunnel: [w547 w555] -> w537
          tunnel: w536 -> [_ w554]
          tunnel: [w546 w553] -> w535
          tunnel: w534 -> [w546 w552]
          tunnel: w533 -> [w545 w551]
          tunnel: [w545 w550] -> w532
          tunnel: w531 -> [_ w549]
          frame False {
          }
          frame True {
            n176 = call "Select Device.vi"("Devices"=w559) -> ("Cancelled?"=w561:bool, "Device out"=w560:i32)  [unwired: 9 in]
            n177 = property on="Open camera" class="Bool (strict)"("Value"=FALSE ("Open device")) -> ()  [unwired: 2 in, 2 out]
            n178 = case shown="False" w561 {
              tunnel: w560 -> [w566 _]
              tunnel: w559 -> [_ _]
              tunnel: w558 -> [w572 w576]
              tunnel: w557 -> [w571 w575]
              tunnel: [w572 w576] -> w556
              tunnel: [w571 w575] -> w555
              tunnel: w554 -> [_ _]
              tunnel: [w570 w574] -> w553
              tunnel: w552 -> [w570 w574]
              tunnel: w551 -> [w569 w573]
              tunnel: [w569 w573] -> w550
              tunnel: w549 -> [w568 _]
              frame False {
                w567 = T3 {"Driver"=0, "Camera settings"=variant, "Update camera table"=TRUE}  # Open camera
                n179 = Bundle By Name(cluster=w567, "Driver"=w566, "Camera settings"=variant, "Update camera table"=TRUE) -> (w565:T3)
                n180 = Generate User Event(user event=w568, event data cluster=w565) -> ()  [unwired: 2 in, 2 out]
              }
              frame True {
              }
            }
          }
        }
      }
      event User Event {
        w592 = 0.01  # Default exposure
        n181 = event-data() -> ("Driver"=w586:i32, "Camera settings"=w585:variant, "Update camera table"=w583:bool)  [unwired: 1 in]
        n182 = Index Array(array=w617, index=w586) -> (element=w610:path)
        n183 = call <vilib>:"Set Busy.vi"() -> ("error out"=w596:errorcluster)  [unwired: 10 in, 1 out]
        n184 = Index Array(array=w579, index=0) -> (element=w578:refnum<vi>)
        n185 = Open VI Reference(type specifier VI Refnum (for type only)=w578, vi path=w610, options=256, error in (no error)=w596) -> (vi reference=w589:refnum<vi>, error out=w606:errorcluster)  [unwired: 2 in]
        n186 = disable-structure shown="Enabled" {
          disable-tunnel: w589 -> [w626 w627]
          disable-tunnel: [w625 w627] -> w588
          frame Disabled {
            n187 = invoke class="VI (strict)" method="FP.Open"(reference=w626, "Activate"=TRUE ("Activate?"), "State"=T8."Standard") -> (reference out=w625:refnum<vi>)  [unwired: 2 in, 4 out]
          }
          frame Enabled {
            # "Don't auto-open front panel\n(for debugging)"
          }
        }
        n188 = call-by-ref "?"(reference=w588, error in=w606, "Operation"=T7."Initialize", "Camera-specific in"=w585, "Exposure time (s)"=w592) -> (reference out=w609:refnum<vi>, error out=w605:errorcluster, "Camera-specific out"=w607:variant, "Status"=w608:T10)  [unwired: 11 in]
        n189 = Unbundle By Name(w608) -> ("System OK?"=w590:bool, "Current exposure"=w597:dbl)
        n190 = call-by-ref "?"(reference=w609, error in=w605, "Operation"=T7."Set capture mode", "Camera-specific in"=w607, "Capture mode"=enum16{"Single frame", "Sequence"}."Single frame") -> (reference out=w602:refnum<vi>, error out=w581:errorcluster, "Camera-specific out"=w601:variant, "Status"=w604:T10)  [unwired: 11 in]
        n191 = call <vilib>:"Unset Busy.vi"("error in (no error)"=w581) -> ("error out"=w603:errorcluster)  [unwired: 10 in]
        n192 = Unbundle By Name(w604) -> ("System OK?"=w593:bool)
        n193 = Unbundle By Name(w603) -> ("status"=w594:bool)
        n194 = Not(x=w594) -> (.not. x?=w595:bool)
        n195 = Compound Arithmetic op=AND(w595, w593, w590) -> (w582:bool)
        n196 = And(x=w582, y=w583) -> (x .and. y?=w584:bool)
        n197 = case shown="True" w584 {
          tunnel: w597 -> [_ w646]
          tunnel: w615 -> [w630 w644]
          tunnel: [w630 w643] -> w616
          tunnel: w587 -> [_ w641]
          tunnel: w586 -> [_ w640]
          tunnel: w582 -> [w629 _]
          tunnel: w581 -> [w628 _]
          frame False {
            n198 = case shown="False" w629 {
              tunnel: w628 -> [w634 _]
              frame False {
                w631 = T11 0 items=["no dialog", "OK message", "continue or stop message", "OK message + warnings", "continue/stop + warnings"] ("type of dialog (OK msg:1)")
                n199 = call <vilib>:"Simple Error Handler.vi"("type of dialog (OK msg:1)"=w631, "error in (no error)"=w634) -> ("error?"=w633:bool, "message"=w632:string)  [unwired: 3 in, 3 out]
                n200 = Concatenate Strings("Error loading camera:\n" ("message"), w632) -> (w635:string)
                n201 = Select(t=w635, s=w633, f="Error loading camera" ("message")) -> (s? t:f=w638:string)
                n202 = One Button Dialog(message=w638) -> ()  [unwired: 1 in, 1 out]
              }
              frame True {
              }
            }
          }
          frame True {
            n203 = property on="Camera settings table" class="MCListbox (strict)"() -> ("ItemNames"=w649:string[][])  [unwired: 2 in, 2 out]
            n204 = Index Array(array=w641, index=w640) -> (element=w639:string)
            n205 = Number To Fractional String(number=w646, precision (6)=i16 3) -> (F-format string=w645:string)  [unwired: 2 in]
            n206 = for {
              N: 1 -> [_]
              shift-right: [w657] -> w648
              shift-left: w649 -> [w656]
              tunnel: w639 -> [w664]
              shift-right: [w653] -> w643
              shift-left: w644 -> [w654]
              tunnel: w645 -> [w658]
              n207 = Equal?(x=w664, y=w656) -> (x = y?=w666:bool[][])
              n208 = Or Array Elements(Boolean array=w666) -> (logical OR=w665:bool)
              n209 = case shown="True" w665 {
                tunnel: w656 -> [_ w672]
                tunnel: w664 -> [w669 w671]
                tunnel: [w669 w670] -> w663
                frame False {
                }
                frame True {
                  n210 = while {
                    tunnel: w672 -> [w679]
                    tunnel: w671 -> [w674]
                    tunnel: [w678] -> w670
                    i -> [w681]
                    stop <- w676 continue-if-true
                    n211 = call <vilib>:"Space Constant.vi"() -> ("String"=w673:string)
                    n212 = Increment(x=w681) -> (x+1=w675:i32)
                    n213 = Number To Decimal String(number=w675) -> (decimal integer string=w680:string)  [unwired: 1 in]
                    n214 = Concatenate Strings(w674, w673, w680) -> (w678:string)
                    n215 = Equal?(x=w678, y=w679) -> (x = y?=w677:bool[][])
                    n216 = Or Array Elements(Boolean array=w677) -> (logical OR=w676:bool)
                  }
                }
              }
              n217 = Build Array(w663, w658, "1" ("element"), "NaN °C" ("element"), "Yes" ("element")) -> (w655:string[])
              n218 = Array Size(array=w656) -> (size(s)=w668:i32[])
              n219 = Index Array(array=w668, index=0) -> (element=w652:i32)
              n220 = Bundle By Name(cluster=T4 {"Row"=0, "Column"=0} ("Active Cell:Active Cell"), "Row"=w652, "Column"=0 ("Row")) -> (w661:T4)
              n221 = Build Array (concatenate)(w654, w652) -> (w653:i32[])
              n222 = Build Array (concatenate)(w656, w655) -> (w657:string[][])
              n223 = property on="Camera settings table" class="MCListbox (strict)"("ActiveCell"=w661) -> ()  [unwired: 2 in, 2 out]
            }
            n224 = property on="Camera settings table" class="MCListbox (strict)"("ItemNames"=w648) -> ()  [unwired: 2 in, 2 out]
          }
        }
        n225 = case shown="True" w582 {
          tunnel: w602 -> [w687 w706]
          tunnel: w601 -> [w686 w709]
          tunnel: w620 -> [w688 w711]
          tunnel: w579 -> [w689 w708]
          tunnel: [w688 w710] -> w619
          tunnel: [w689 w707] -> w618
          tunnel: w614 -> [w682 w704]
          tunnel: [w682 w690] -> w613
          tunnel: w612 -> [_ w697]
          tunnel: w611 -> [_ w696]
          frame False {
            n226 = call-by-ref "?"(reference=w687, "Operation"=T9."Shut down", "Camera-specific in"=w686) -> (reference out=w684:refnum<vi>)  [unwired: 13 in, 3 out]
            n227 = property on="Status" class="Str"("Value"="Camera error - closing connection" ("Status")) -> ()  [unwired: 2 in, 2 out]
            n228 = Close Reference(reference=w684) -> ()  [unwired: 1 in, 1 out]
          }
          frame True {
            w695 = u16 1 items=["Shutdown", "Update image references"]  # Operation
            w705 = T12 7 items=["Grayscale (U8)", "Grayscale (I16)", "Grayscale (SGL)", "Complex (CSG)", "RGB (U32)", "HSL (U32)", "RGB (U64)", "Grayscale (U16)"] ("Image Type")
            n229 = feedback #3(0) -> (w699:i32)
            n230 = Increment(x=w699) -> (x+1=w691:i32)
            n231 = feedback-in #3(w691) -> ()
            n232 = Number To Decimal String(number=w691) -> (decimal integer string=w698:string)  [unwired: 1 in]
            n233 = Build Array (concatenate)(w711, w709) -> (w710:variant[])
            n234 = Build Array (concatenate)(w708, w706) -> (w707:refnum<vi>[])
            n235 = Concatenate Strings("Camera Image " ("Image Name"), w698) -> (w701:string)
            n236 = call "IMAQ Create"("Image Name"=w701, "Image Type"=w705) -> ("New Image"=w703:T1)  [unwired: 3 in, 1 out]
            n237 = Build Array (concatenate)(w704, w703) -> (w690:T1[])
            n238 = To Variant(anything=w690) -> (Variant=w692:variant)
            n239 = Bundle("Operation"=w695, "Variant"=w692) -> (w694:cluster{"Operation":u16, "Variant":variant})  [unwired: 1 in]
            n240 = To Variant(anything=w694) -> (Variant=w693:variant)
            n241 = Generate User Event(user event=w697, event data cluster=w690) -> ()  [unwired: 2 in, 2 out]
            n242 = Enqueue Element(queue=w696, element=w693) -> ()  [unwired: 2 in, 3 out]
          }
        }
      }
      event "Close camera": Value Change {
        n243 = event-data() -> ("NewVal"=w725:bool)  [unwired: 1 in]
        n244 = case shown="True" w725 {
          tunnel: w723 -> [_ _]
          tunnel: w722 -> [w730 w739]
          tunnel: w720 -> [w729 w740]
          tunnel: [w730 w735] -> w721
          tunnel: [w729 w736] -> w719
          tunnel: [w728 w737] -> w718
          tunnel: w717 -> [w728 w738]
          tunnel: w716 -> [w727 w734]
          tunnel: [w727 w733] -> w715
          tunnel: w714 -> [_ w732]
          tunnel: w713 -> [_ w731]
          frame False {
          }
          frame True {
            n245 = property on="Camera settings table" class="MCListbox (strict)"() -> ("Value"=w741:i32, "ItemNames"=w744:string[][])  [unwired: 2 in, 2 out]
            n246 = Greater Or Equal To 0?(x=w741) -> (x >= 0?=w742:bool)
            n247 = case shown="True" w742 {
              tunnel: w744 -> [_ w755]
              tunnel: [FALSE ("T button?") w750] -> w743
              tunnel: w741 -> [_ w749]
              frame False {
                n248 = One Button Dialog(message="Please select a valid device") -> ()  [unwired: 1 in, 1 out]
              }
              frame True {
                n249 = Index Array(array=w755, index (row)=w749, index (col)=0 ("disabled index (col)")) -> (element=w752:string)
                n250 = Concatenate Strings("Close camera ", w752, "?" ("string")) -> (w748:string)
                n251 = Two Button Dialog(message=w748) -> (T button?=w750:bool)  [unwired: 2 in]
              }
            }
            n252 = property on="Close camera" class="Bool (strict)"("Value"=FALSE ("Open device")) -> ()  [unwired: 2 in, 2 out]
            n253 = case shown="True" w743 {
              tunnel: [w759 w788] -> w736
              tunnel: w740 -> [w759 w789]
              tunnel: [w758 w786] -> w735
              tunnel: w739 -> [w758 w787]
              tunnel: [w757 w761] -> w737
              tunnel: w738 -> [w757 w785]
              tunnel: w741 -> [_ w790]
              tunnel: w734 -> [w756 w771]
              tunnel: [w756 w760] -> w733
              tunnel: w732 -> [_ w767]
              tunnel: w731 -> [_ w762]
              frame False {
              }
              frame True {
                w763 = u16 1 items=["Shutdown", "Update image references"]  # Operation
                w779 = 0 ("index")
                w770 = 1 ("length")
                n254 = Index Array(array=w785, index=w790) -> (element=w769:i32)
                n255 = for {
                  tunnel: w769 -> [w793]
                  shift-right: [w796] -> w761
                  shift-left: i32[] [] -> [w797]
                  tunnel: w785 -> [w794] mode=indexing
                  tunnel: [w792] -> w775
                  i -> [w792]
                  n256 = Equal?(x=w793, y=w794) -> (x = y?=w795:bool)
                  n257 = case shown="False" w795 {
                    tunnel: w797 -> [w804 w809]
                    tunnel: [w803 w809] -> w796
                    tunnel: w794 -> [w799 _]
                    tunnel: w793 -> [w798 _]
                    tunnel: w792 -> [_ w805]
                    frame False {
                      n258 = Less?(x=w799, y=w798) -> (x < y?=w800:bool)
                      n259 = Decrement(x=w799) -> (x-1=w801:i32)
                      n260 = Select(t=w799, s=w800, f=w801) -> (s? t:f=w802:i32)
                      n261 = Build Array (concatenate)(w804, w802) -> (w803:i32[])
                    }
                    frame True {
                      n262 = property on="Camera settings table" class="MCListbox (strict)"() -> ("ItemNames"=w808:string[][])  [unwired: 2 in, 2 out]
                      n263 = Delete From Array(array=w808, length=1, index (row)=w805) -> (array with subset deleted=w807:string[][])  [unwired: 1 in, 1 out]
                      n264 = property on="Camera settings table" class="MCListbox (strict)"("ItemNames"=w807) -> ()  [unwired: 2 in, 2 out]
                    }
                  }
                }
                n265 = Bundle(w775, 0) -> (w773:cluster{i32, i32})  [unwired: 1 in]
                n266 = property on="Camera settings table" class="MCListbox (strict)"("ActiveCell"=w773, "CellBG"=u32 16777215) -> ()  [unwired: 2 in, 2 out]
                n267 = Delete From Array(array=w789, length=w770, index=w769) -> (deleted portion=w781:refnum<vi>[], array with subset deleted=w788:refnum<vi>[])
                n268 = Delete From Array(array=w787, length=w770, index=w769) -> (deleted portion=w782:variant[], array with subset deleted=w786:variant[])
                n269 = Delete From Array(array=w771, length=w770, index=w769) -> (deleted portion=w768:T1[], array with subset deleted=w760:T1[])
                n270 = for {
                  tunnel: w768 -> [w791] mode=indexing
                  n271 = call "IMAQ Dispose"("Image"=w791) -> ()  [unwired: 5 in, 1 out]
                }
                n272 = Index Array(array=w781, index=w779) -> (element=w778:refnum<vi>)
                n273 = Index Array(array=w782, index=w779) -> (element=w780:variant)
                n274 = call-by-ref "?"(reference=w778, "Operation"=T7."Shut down", "Camera-specific in"=w780) -> (reference out=w783:refnum<vi>, error out=w784:errorcluster)  [unwired: 13 in, 2 out]
                n275 = Close Reference(reference=w783, error in (no error)=w784) -> ()  [unwired: 1 out]
                n276 = To Variant(anything=w760) -> (Variant=w766:variant)
                n277 = Bundle("Operation"=w763, "Variant"=w766) -> (w764:cluster{"Operation":u16, "Variant":variant})  [unwired: 1 in]
                n278 = Generate User Event(user event=w767, event data cluster=w760) -> ()  [unwired: 2 in, 2 out]
                n279 = To Variant(anything=w764) -> (Variant=w765:variant)
                n280 = Enqueue Element(queue=w762, element=w765) -> ()  [unwired: 2 in, 3 out]
              }
            }
          }
        }
      }
      event "Camera settings": Value Change {
        n281 = event-data() -> ("NewVal"=w817:bool)  [unwired: 1 in]
        n282 = case shown="True" w817 {
          tunnel: w820 -> [w822 w832]
          tunnel: [w822 w833] -> w818
          tunnel: [w821 w831] -> w816
          tunnel: w815 -> [w821 w830]
          tunnel: w813 -> [_ w827]
          tunnel: w811 -> [_ w824]
          tunnel: w810 -> [_ w823]
          frame False {
          }
          frame True {
            n283 = property on="Camera settings table" class="MCListbox (strict)"() -> ("Value"=w826:i32)  [unwired: 2 in, 2 out]
            n284 = Greater Or Equal To 0?(x=w826) -> (x >= 0?=w829:bool)
            n285 = property on="Camera settings" class="Bool (strict)"("Value"=FALSE ("Camera settings")) -> ()  [unwired: 2 in, 2 out]
            n286 = case shown="False" w829 {
              selector: w829 -> [_ w865]
              tunnel: [FALSE ("T button?") w865] -> w828
              frame False {
                n287 = One Button Dialog(message="Please select a valid camera") -> ()  [unwired: 1 in, 1 out]
              }
              frame True {
              }
            }
            n288 = Index Array(array=w827, index=w826) -> (element=w825:i32)
            n289 = case shown="True" w828 {
              tunnel: [w835 w853] -> w833
              tunnel: w832 -> [w835 w852]
              tunnel: [w836 w850] -> w831
              tunnel: w830 -> [w836 w849]
              tunnel: w825 -> [_ w842]
              tunnel: w824 -> [_ w843]
              tunnel: w823 -> [_ w840]
              frame False {
              }
              frame True {
                n290 = Index Array(array=w843, index=w842) -> (element=w841:T1)
                n291 = Index Array(array=w849, index=w842) -> (element=w851:variant)
                n292 = Index Array(array=w852, index=w842) -> (element=w854:refnum<vi>)
                n293 = Bundle("New Image"=w841, "Image"=w840, 10.0) -> (w838:cluster{"New Image":T1, "Image":refnum<vi>, dbl})  [unwired: 1 in]
                n294 = To Variant(anything=w838) -> (Variant=w837:variant)
                n295 = call-by-ref "?"(reference=w854, "Operation"=T7."Other settings", "Camera-specific in"=w851, "Image in"=w837) -> (reference out=w847:refnum<vi>, "Camera-specific out"=w845:variant)  [unwired: 12 in, 2 out]
                n296 = disable-structure shown="Enabled" {
                  disable-tunnel: w847 -> [w860 w862]
                  disable-tunnel: [w859 w862] -> w846
                  disable-tunnel: w845 -> [w858 w861]
                  disable-tunnel: [w857 w861] -> w844
                  frame Disabled {
                    n297 = call-by-ref "?"(reference=w860, "Operation"=T9."Set capture mode", "Camera-specific in"=w858, "Capture mode"=enum16{"Single frame", "Sequence"}."Single frame") -> (reference out=w859:refnum<vi>, "Camera-specific out"=w857:variant)  [unwired: 12 in, 2 out]
                  }
                  frame Enabled {
                    # "Because some cameras need to reinitialize. Do it yourself!!"
                  }
                }
                n298 = Replace Array Subset(array=w852, new element=w846, index=w842) -> (w853:refnum<vi>[])
                n299 = Replace Array Subset(array=w849, new element=w844, index=w842) -> (w850:variant[])
              }
            }
          }
        }
      }
      event "Camera settings table": Double Click {
        w867 = "Yes"
        n300 = event-data() -> ("Coords"=w897:T13)  [unwired: 1 in]
        n301 = invoke on="Camera settings table" class="MCListbox (strict)" method="Point To Row Column"("Point"=w897) -> ("CellPosition"=w896:T4)  [unwired: 6 in, 6 out]
        n302 = property on="Camera settings table" class="MCListbox (strict)"() -> ("ItemNames"=w884:string[][])  [unwired: 2 in, 2 out]
        n303 = Unbundle By Name(w896) -> ("Row"=w870:i32, "Column"=w886:i32)
        n304 = Index Array(array=w884, index (row) #1=w870, index (col) #1=0 ("disabled index (col)"), index (row) #2=w870, index (col) #2=1 ("disabled index (col)"), index (row) #3=w870, index (col) #3=2 ("disabled index (col)"), index (row) #4=w870, index (col) #4=4 ("index (col)")) -> (element #1=w889:string, element #2=w887:string, element #3=w892:string, element #4=w869:string)
        n305 = Array Size(array=w878) -> (size(s)=w877:i32)
        n306 = Equal?(x=w869, y=w867) -> (x = y?=w868:bool)
        n307 = Less?(x=w870, y=w877) -> (x < y?=w876:bool)
        n308 = Not Equal?(x=w870, y=-1) -> (x != y?=w875:bool)
        n309 = Fract/Exp String To Number(string=w887, default (0 dbl)=0.0 ("default (0 I32)")) -> (number=w885:dbl)  [unwired: 2 in, 1 out]
        n310 = And(x=w876, y=w875) -> (x .and. y?=w873:bool)
        n311 = Fract/Exp String To Number(string=w892, default (0 dbl)=0.0 ("default (0 I32)")) -> (number=w890:dbl)  [unwired: 2 in, 1 out]
        n312 = case "Don't accept clicks on things that aren't cameras" shown="True" w873 {
          tunnel: w890 -> [_ w916]
          tunnel: w889 -> [_ w915]
          tunnel: w886 -> [_ w914]
          tunnel: w885 -> [_ w913]
          tunnel: w884 -> [w900 w912]
          tunnel: w883 -> [_ w911]
          tunnel: [w902 w910] -> w882
          tunnel: w881 -> [w902 w909]
          tunnel: [w901 w908] -> w880
          tunnel: [w900 w907] -> w879
          tunnel: w878 -> [w901 w906]
          tunnel: w870 -> [_ w905]
          tunnel: w868 -> [_ w904]
          tunnel: w867 -> [_ w903]
          frame False {
          }
          frame True {
            n313 = case "Column clicked on" shown="1" w914 {
              tunnel: w905 -> [_ w931 w968 w990]
              tunnel: w915 -> [_ w930 w967 _]
              tunnel: w916 -> [_ _ w957 _]
              tunnel: w913 -> [_ w927 _ _]
              tunnel: w912 -> [w917 w923 w961 w992]
              tunnel: w911 -> [_ w926 w964 _]
              tunnel: w906 -> [w918 w925 w963 w994]
              tunnel: w909 -> [w919 w924 w962 w995]
              tunnel: [w919 w922 w960 w995] -> w910
              tunnel: [w918 w921 w959 w994] -> w908
              tunnel: [w917 w920 w958 w991] -> w907
              tunnel: w904 -> [_ _ _ w988]
              tunnel: w903 -> [_ _ _ w987]
              frame 0, Default {
                # "Name"
              }
              frame 1 {
                # "Exposure"
                n314 = Concatenate Strings(w930, " Exposure" ("string")) -> (w929:string)
                n315 = call "ChangeValuePopup.vi"("Device description"=w929, "Initial value"=w927) -> ("Device value"=w932:dbl, "OK"=w933:bool)  [unwired: 15 in, 1 out]
                n316 = case shown="True" w933 {
                  tunnel: w932 -> [_ w942]
                  tunnel: w931 -> [_ w944]
                  tunnel: w926 -> [_ w952]
                  tunnel: w925 -> [w936 w954]
                  tunnel: w924 -> [w935 w956]
                  tunnel: w923 -> [w934 w945]
                  tunnel: [w935 w955] -> w922
                  tunnel: [w936 w953] -> w921
                  tunnel: [w934 w939] -> w920
                  frame False {
                  }
                  frame True {
                    n317 = Index Array(array=w952, index=w944) -> (element=w951:i32)
                    n318 = Index Array(array=w956, index=w951) -> (element=w948:variant)
                    n319 = Index Array(array=w954, index=w951) -> (element=w950:refnum<vi>)
                    n320 = call-by-ref "?"(reference=w950, "Operation"=T7."Set exposure", "Camera-specific in"=w948, "Exposure time (s)"=w942) -> (reference out=w949:refnum<vi>, "Camera-specific out"=w947:variant, "Status"=w938:T10)  [unwired: 12 in, 1 out]
                    n321 = Unbundle By Name(w938) -> ("Current exposure"=w937:dbl)
                    n322 = Number To Exponential String(number=w937, precision (6)=i16 3) -> (E-format string=w940:string)  [unwired: 2 in]
                    n323 = Replace Array Subset(array=w945, new element=w940, index (row)=w944, index (col)=1 ("disabled index (col)")) -> (w939:string[][])
                    n324 = Replace Array Subset(array=w956, new element=w947, index=w951) -> (w955:variant[])
                    n325 = Replace Array Subset(array=w954, new element=w949, index=w951) -> (w953:refnum<vi>[])
                  }
                }
              }
              frame 2 {
                # "Frames per position"
                n326 = Concatenate Strings(w967, " Frames per position" ("string")) -> (w966:string)
                n327 = call "ChangeValuePopup.vi"("Device description"=w966, "Initial value"=w957) -> ("Device value"=w969:dbl, "OK"=w970:bool)  [unwired: 15 in, 1 out]
                n328 = case shown="True" w970 {
                  tunnel: w969 -> [_ w978]
                  tunnel: w968 -> [_ w984]
                  tunnel: w964 -> [_ _]
                  tunnel: w963 -> [w973 w979]
                  tunnel: w962 -> [w972 w980]
                  tunnel: w961 -> [w971 w985]
                  tunnel: [w972 w980] -> w960
                  tunnel: [w973 w979] -> w959
                  tunnel: [w971 w981] -> w958
                  frame False {
                  }
                  frame True {
                    n329 = In Range and Coerce(upper limit=inf, x=w978, lower limit=1.0) -> (coerced(x)=w977:dbl)  [unwired: 1 out]
                    n330 = To Unsigned Long Integer(number=w977) -> (unsigned 32bit integer=w974:u32)
                    n331 = Number To Decimal String(number=w974) -> (decimal integer string=w982:string)  [unwired: 1 in]
                    n332 = Replace Array Subset(array=w985, new element=w982, index (row)=w984, index (col)=2 ("disabled index (col)")) -> (w981:string[][])
                  }
                }
              }
              frame 4 {
                # "Live?"
                n333 = Select(t="No", s=w988, f=w987) -> (s? t:f=w989:string)
                n334 = Replace Array Subset(array=w992, new element=w989, index (row)=w990, index (col)=4 ("disabled index (col)")) -> (w991:string[][])
              }
            }
          }
        }
        n335 = property on="Camera settings table" class="MCListbox (strict)"("ItemNames"=w879) -> ()  [unwired: 2 in, 2 out]
      }
    }
    n336 = feedback-in #1(w137) -> ()
  }
  n337 = Destroy User Event(user event=w27) -> ()  [unwired: 1 in, 1 out]
  n338 = Destroy User Event(user event=w83) -> ()  [unwired: 1 in, 1 out]
  n339 = Destroy User Event(user event=w1) -> ()  [unwired: 1 in, 1 out]
  n340 = Destroy User Event(user event=w23) -> ()  [unwired: 1 in, 1 out]
  n341 = Destroy User Event(user event=w81) -> ()  [unwired: 1 in, 1 out]
  n342 = Obtain Queue(name (unnamed)="Display/panel send data", element data type=w16) -> (queue out=w20:refnum<queue>)  [unwired: 3 in, 2 out]
  n343 = while "Display / UI processing" {
    tunnel: w78 -> [w1011]
    tunnel: [w1008] -> w77
    tunnel: w76 -> [w1008]
    tunnel: w11 -> [w1006]
    tunnel: [w1006] -> w53
    shift-right: [w1005] -> _
    shift-left: T1[] [] ("appended array") -> [w1007]
    tunnel: w44 -> [w1004]
    tunnel: w43 -> [w1003]
    shift-right: [w1000] -> w31
    shift-left: w41 -> [w1002]
    shift-right: [w999] -> w30
    shift-left: w42 -> [w1001]
    tunnel: w40 -> [w998]
    tunnel: w20 -> [w997]
    tunnel: [w997] -> w19
    tunnel: w10 -> [w996]
    tunnel: [w996] -> w9
    stop <- w1010 stop-if-true
    n344 = event shown="[2] <Update image references>: User Event" {
      selector: w1011 -> [_ _ _ _]
      dyn-events: _ -> [_ _ _ _]
      timeout: 30 -> [_ _ _ _]
      tunnel: [_ TRUE _ _] -> w1010
      tunnel: w1007 -> [w1014 w1017 _ w1031]
      tunnel: [w1014 w1017 w1020 w1031] -> w1005
      tunnel: w1004 -> [_ _ _ w1032]
      tunnel: w1003 -> [_ _ _ w1033]
      tunnel: w1002 -> [w1013 w1016 w1025 w1027]
      tunnel: w1001 -> [w1012 w1015 w1024 w1026]
      tunnel: [w1013 w1016 w1025 w1035] -> w1000
      tunnel: [w1012 w1015 w1024 w1034] -> w999
      tunnel: w998 -> [_ _ _ w1030]
      tunnel: w997 -> [_ _ w1023 w1028]
      event Timeout {
        n345 = event-data() -> ()  [unwired: 1 in, 3 out]
      }
      event User Event {
        n346 = event-data() -> ()  [unwired: 1 in, 5 out]
      }
      event User Event {
        n347 = event-data() -> ("Update image references"=w1020:T1[])  [unwired: 1 in, 4 out]
        n348 = To Variant(anything=w1020) -> (Variant=w1019:variant)
        n349 = Bundle(enum16{"Image references", "Positions"}."Image references", "Variant"=w1019) -> (w1021:T14)  [unwired: 1 in]
        n350 = Enqueue Element(queue=w1023, element=w1021) -> ()  [unwired: 2 in, 3 out]
      }
      event "Display and panel": Value Change {
        w1036 = 128
        n351 = event-data() -> ("NewVal"=w1029:i32)  [unwired: 1 in]
        n352 = Index Array(array=w1030, index=w1029) -> (element=w1060:path)
        n353 = invoke class="VI (strict)" method="Abort VI"(reference=w1026) -> (reference out=w1044:refnum<vi>, error out=w1046:errorcluster)  [unwired: 2 in, 1 out]
        n354 = Path To String(path=w1060) -> (string=w1059:string)
        n355 = String Length(string=w1059) -> (length=w1058:i32)
        n356 = invoke class="VI (strict)" method="Abort VI"(reference=w1027) -> (reference out=w1049:refnum<vi>, error out=w1051:errorcluster)  [unwired: 2 in, 1 out]
        n357 = Subtract(x=w1058, y=11) -> (x-y=w1057:i32)
        n358 = String Subset(string=w1059, offset (0)=0, length (rest)=w1057) -> (substring=w1056:string)
        n359 = Concatenate Strings(w1056, "_Panel.vi" ("string")) -> (w1055:string)
        n360 = String To Path(string=w1055) -> (path=w1054:path)
        n361 = call <vilib>:"Clear Errors.vi"("error in (no error)"=w1046) -> ("error out"=w1045:errorcluster)  [unwired: 5 in, 1 out]
        n362 = Close Reference(reference=w1044) -> (error out=w1047:errorcluster)  [unwired: 1 in]
        n363 = Close Reference(reference=w1049) -> (error out=w1048:errorcluster)  [unwired: 1 in]
        n364 = invoke on="Control Sub Panel" class="SubPnl" method="Remove VI"(error in=w1045) -> (error out=w1042:errorcluster)  [unwired: 2 in, 2 out]
        n365 = call <vilib>:"Clear Errors.vi"("error in (no error)"=w1051) -> ("error out"=w1050:errorcluster)  [unwired: 5 in, 1 out]
        n366 = call <vilib>:"Clear Errors.vi"("error in (no error)"=w1047) -> ("error out"=w1043:errorcluster)  [unwired: 5 in, 1 out]
        n367 = call <vilib>:"Clear Errors.vi"("error in (no error)"=w1048) -> ("error out"=w1040:errorcluster)  [unwired: 5 in, 1 out]
        n368 = Open VI Reference(type specifier VI Refnum (for type only)=w1027, vi path=w1060, options=w1036, error in (no error)=w1040) -> (vi reference=w1053:refnum<vi>)  [unwired: 2 in, 1 out]
        n369 = Open VI Reference(type specifier VI Refnum (for type only)=w1026, vi path=w1054, options=w1036, error in (no error)=w1043) -> (vi reference=w1052:refnum<vi>)  [unwired: 2 in, 1 out]
        n370 = invoke on="Display Sub Panel" class="SubPnl" method="Remove VI"(error in=w1050) -> (error out=w1041:errorcluster)  [unwired: 2 in, 2 out]
        n371 = invoke on="Control Sub Panel" class="SubPnl" method="Insert VI"(error in=w1042, "VI Ref"=w1052) -> ()  [unwired: 2 in, 4 out]
        n372 = invoke on="Display Sub Panel" class="SubPnl" method="Insert VI"(error in=w1041, "VI Ref"=w1053) -> ()  [unwired: 2 in, 4 out]
        n373 = call-by-ref "Start Asynchronous Call"(reference=w1053, "Input data"=w1031, "Link out"=w1032, "Link in"=w1033) -> (reference out=w1035:refnum<vi>)  [unwired: 10 in, 1 out]
        n374 = call-by-ref "Start Asynchronous Call"(reference=w1052, "Data in"=w1028, "Link out"=w1033, "Link in"=w1032) -> (reference out=w1034:refnum<vi>)  [unwired: 10 in, 1 out]
      }
    }
  }
  n375 = Destroy User Event(user event=w9) -> ()  [unwired: 1 in, 1 out]
  n376 = Destroy User Event(user event=w53) -> ()  [unwired: 1 in, 1 out]
  n377 = Destroy User Event(user event=w77) -> ()  [unwired: 1 in, 1 out]
  n378 = Release Queue(queue=w19) -> ()  [unwired: 2 in, 3 out]
  n379 = Release Queue(queue=w57) -> ()  [unwired: 2 in, 3 out]
  n380 = Release Queue(queue=w56) -> ()  [unwired: 2 in, 3 out]
  n381 = invoke class="VI (strict)" method="Abort VI"(reference=w30) -> (reference out=w39:refnum<vi>, error out=w37:errorcluster)  [unwired: 2 in, 1 out]
  n382 = invoke class="VI (strict)" method="Abort VI"(reference=w31) -> (reference out=w34:refnum<vi>, error out=w32:errorcluster)  [unwired: 2 in, 1 out]
  n383 = call <vilib>:"Clear Errors.vi"("error in (no error)"=w37) -> ("error out"=w38:errorcluster)  [unwired: 5 in, 1 out]
  n384 = Close Reference(reference=w34) -> (error out=w35:errorcluster)  [unwired: 1 in]
  n385 = Close Reference(reference=w39) -> (error out=w36:errorcluster)  [unwired: 1 in]
  n386 = call <vilib>:"Clear Errors.vi"("error in (no error)"=w32) -> ("error out"=w33:errorcluster)  [unwired: 5 in, 1 out]
  n387 = invoke on="Control Sub Panel" class="SubPnl" method="Remove VI"(error in=w38) -> ()  [unwired: 2 in, 3 out]
  n388 = call <vilib>:"Clear Errors.vi"("error in (no error)"=w35) -> ()  [unwired: 5 in, 2 out]
  n389 = call <vilib>:"Clear Errors.vi"("error in (no error)"=w36) -> ()  [unwired: 5 in, 2 out]
  n390 = Not A Number/Path/Refnum?(number/path/refnum=w14) -> (NaN/Path/Refnum?=w13:bool)
  n391 = invoke on="Display Sub Panel" class="SubPnl" method="Remove VI"(error in=w33) -> ()  [unwired: 2 in, 3 out]
  n392 = for {
    tunnel: w54 -> [w1061] mode=indexing
    n393 = call "IMAQ Dispose"("Image"=w1061) -> ()  [unwired: 5 in, 1 out]
  }
  n394 = case shown="False" w13 {
    tunnel: w14 -> [w1062 _]
    frame False {
      n395 = Close Reference(reference=w1062) -> ()  [unwired: 1 in, 1 out]
    }
    frame True {
    }
  }
  n396 = for {
    tunnel: w87 -> [w1070] mode=indexing
    tunnel: w86 -> [w1068] mode=indexing
    border: 0 -> [_]
    n397 = call-by-ref "?"(reference=w1070, "Operation"=T7."Shut down", "Camera-specific in"=w1068) -> (reference out=w1071:refnum<vi>, error out=w1072:errorcluster)  [unwired: 13 in, 2 out]
    n398 = Close Reference(reference=w1071, error in (no error)=w1072) -> ()  [unwired: 1 out]
    n399 = feedback #4() -> (w1063:i32)
    n400 = Increment(x=w1063) -> (x+1=w1067:i32)
    n401 = feedback-in #4(w1067) -> ()
    n402 = Bundle(w1063, 0) -> (w1065:cluster{i32, i32})  [unwired: 1 in]
    n403 = property on="Camera settings table" class="MCListbox (strict)"("ActiveCell"=w1065, "CellBG"=u32 16777215) -> ()  [unwired: 2 in, 2 out]
  }
